vi "Demo Seq Tester.vi"() -> ()   [LabVIEW 2014]
uses:
  <vilib>/Utility/miscctls.llb/LVRowAndColumnTypeDef.ctl
  TypeDefs/STEP Display.ctl
  Mimico Display/TypeDefs/Mimic Data.ctl
  Mimico Display/TypeDefs/BG Image.ctl
  Mimico Display/TypeDefs/mObject.ctl
  SeqLoop/TypeDefs/Sequence.ctl
  SeqLoop/Classes/STEP/STEP.lvclass
  SeqLoop/TypeDefs/LogicParsedExpression.ctl
  SeqLoop/TypeDefs/HW InOut MAP.ctl
  SeqLoop/TypeDefs/Program.ctl
  APIs/Data Queue/Control Data Cluster.ctl
  SEQ Monitoring Global Variables.vi
  DO Monitoring Global Variables.vi
  APIs/Message Queue/Enqueue Message (Single).vi
  APIs/Message Queue/WINFAS 2 Message Queue.lvlib
  SeqLoop/SeqLoop.lvlib
  Mimico Display/Mimico Display.lvlib
  APIs/Data Queue/WINFAS 2 Data Queue.lvlib
panel:
  out "Current Prog Name":string caption="Info"
  out "Current Prog Info":string caption="Info"
  in  "MIMIC":bool
  in  "SEC":bool
  in  "HOME":bool
  in  "Tab Control":enum32{"HOME", "SEC", "MIMIC", "MESSAGE"}(tab)=enum."SEC"
  in  "New Cfg":bool
  in  "Open Cfg":bool
  in  "Save Cfg":bool
  in  "New Prog":bool
  in  "Delete Prog":bool
  in  "Config Prog":bool
  in  "I/O Config":bool
  in  "Editor de Programas":i32(listbox)=-1 caption="Secuencia"
  out "Current Sequence":string[][](table)
  in  "Angle":sgl(knob) scale=-720.0..720.0
  in  "Start Sec A-Z":bool
  in  "Start Sec Ciclo":bool
  in  "Tab Control HardW":enum32{"Hw 1", "Hw 2", "Hw 3", "Hw 4", "Hw 5"}(tab)
  in  "Conf In":T1
  in  "Conf In 2":T1
  in  "Conf In 3":T1
  in  "Conf In 4":T1
  in  "Conf In 5":T1
  in  "OutPuts":T2(tab)
  out "View Out":T3
  out "View Out 2":T3
  out "View Out 3":T3
  out "View Out 4":T3
  out "View Out 5":T3
  out "Error":bool
  out "Alarma":bool
  in  "Start Sec Special":bool
  out "Show Main Error&Alarm":string[][](table)
  out "Acept":bool
  out "Alarms Message":string
  out "Error Message":string
  out "Operator Message":string
  out "Mimic":picture
  out "MATH":string
  out "HWAsync 10":string
  out "HWAsync 9":string
  out "HWAsync 8":string
  out "HWAsync 7":string
  out "HWAsync 6":string
  out "HWAsync 5":string
  out "HWAsync 4":string
  out "HWAsync 3":string
  out "HWAsync 2":string
  out "HWAsync 1":string
  out "HWSync 5":string
  out "DO 5":bool[](array[boolean]) caption="DO-HWSync 5 -->"
  out "HWSync 4":string
  out "DO 4":bool[](array[boolean]) caption="DO-HWSync 4 -->"
  out "HWSync 3":string
  out "DO 3":bool[](array[boolean]) caption="DO-HWSync 3 -->"
  out "HWSync 2":string
  out "DO 2":bool[](array[boolean]) caption="DO-HWSync 2 -->"
  out "HWSync 1":string
  out "DO 1":bool[](array[boolean]) caption="DO-HWSync 1 -->"
  in  "MESSAGE":bool
  in  "error in (no error)":errorcluster
  in  "Tab Control 2":enum32{"HOME", "PIC", "TAB"}(tab)=enum."PIC"
  out "Mimic Small":picture
  out "Cond. Avan.":string[][](table)
  # "DEMO - Secuencial"
  # "Lista de Programas de Medición"
  # "Editor de Programas"
  # "Instrucciones: \n1)Utilice los botones de crear o borrar programa para agregar o borrar la referencia a la \"Lista de Programas de Medición\".\n2)Utilice la opción de configuración de programas para editar o configurar el programa previamente creado o cargado.\n3)Utilice la opción de configuración de I/O para configurar todas las entradas y salidas que se deseen usar."
  # "Configuración"
  # "Secuencia de Ciclo de Medición"
  # "Estado"
  # "Encoder"
  # "Mensaje de Operador:"
  # "Alarmas:"
  # "Dispositivos SINCRONOS"
  # "Módulo MATEMATICO"
  # "Dispositivos ASINCRONOS"
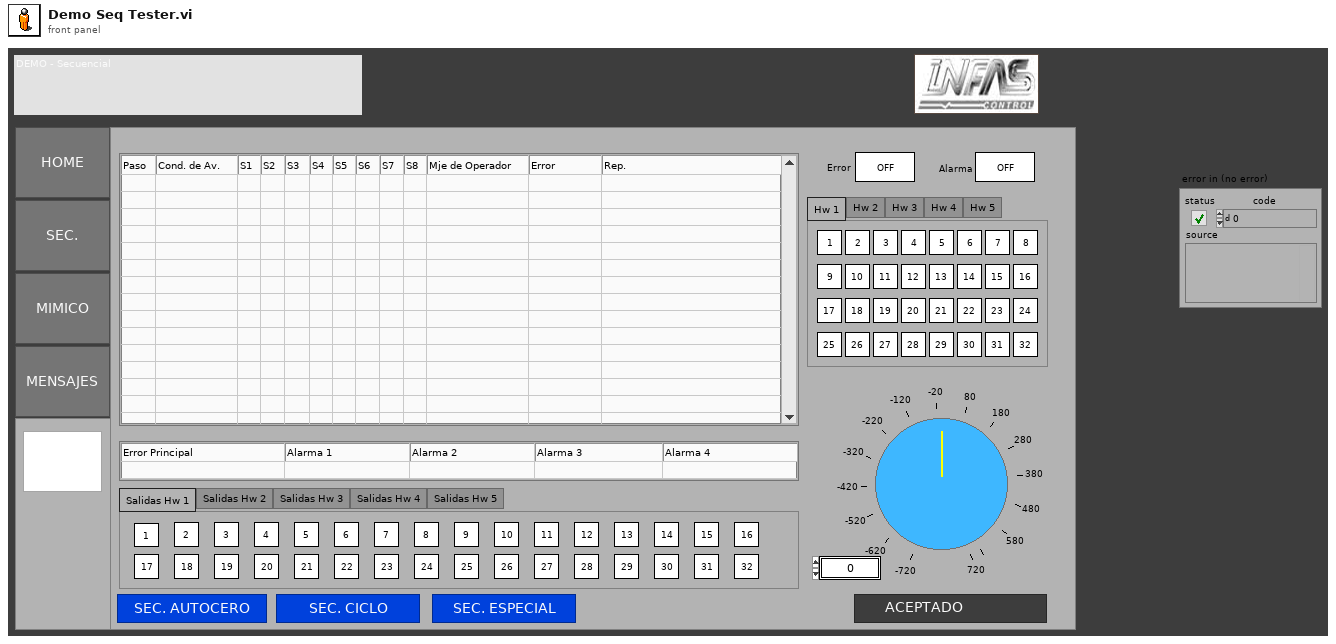
[diagram p1: front panel]
types:
  T1 = cluster{"Boolean 31":bool, "Boolean 2":bool, "Boolean 30":bool, "Boolean 29":bool, "Boolean 28":bool, "Boolean 27":bool, "Boolean 13":bool, "Boolean 14":bool, "Boolean 26":bool, "Boolean 25":bool, "Boolean 24":bool, "Boolean 23":bool, "Boolean 32":bool, "Boolean 1":bool, "Boolean 3":bool, "Boolean 4":bool, "Boolean 5":bool, "Boolean 6":bool, "Boolean 7":bool, "Boolean 8":bool, "Boolean 9":bool, "Boolean 10":bool, "Boolean 11":bool, "Boolean 12":bool, "Boolean 20":bool, "Boolean 18":bool, "Boolean 19":bool, "Boolean 17":bool, "Boolean 16":bool, "Boolean 15":bool, "Boolean 22":bool, "Boolean 21":bool}
  T2 = enum32{"Salidas Hw 1", "Salidas Hw 2", "Salidas Hw 3", "Salidas Hw 4", "Salidas Hw 5"}
  T3 = cluster{"Boolean 36":bool, "Boolean 3":bool, "Boolean 35":bool, "Boolean 34":bool, "Boolean 33":bool, "Boolean 32":bool, "Boolean 16":bool, "Boolean 17":bool, "Boolean 26":bool, "Boolean 25":bool, "Boolean 24":bool, "Boolean 23":bool, "Boolean 37":bool, "Boolean 1":bool, "Boolean 15":bool, "Boolean 4":bool, "Boolean 5":bool, "Boolean 6":bool, "Boolean 7":bool, "Boolean 8":bool, "Boolean 9":bool, "Boolean 10":bool, "Boolean 11":bool, "Boolean 12":bool, "Boolean 38":bool, "Boolean 21":bool, "Boolean 22":bool, "Boolean 20":bool, "Boolean 19":bool, "Boolean 18":bool, "Boolean 40":bool, "Boolean 39":bool}
  T4 = typedef "SeqLoop.lvlib/Sequence.ctl" = cluster{"STEPs":refnum<class "STEP.lvclass">[], "Main Error&Alarm":cluster{"Main Error":T5, "Main Alarm 1":T5, "Main Alarm 2":T5, "Main Alarm 3":T5, "Main Alarm 4":T5}, "STEP Type":refnum<class "STEP.lvclass">}
  T5 = typedef "SeqLoop.lvlib/LogicParsedExpression.ctl" = cluster{"RPN ":string[], "Variables":string[], "Ctes":string[], "Formula":string, "Message":string}
  T6 = cluster{"HWS1":string, "HWS2":string, "HWS3":string, "HWS4":string, "HWS5":string, "MATH":string}
  T7 = enum8{"Enabled", "Disabled", "Disabled and Grayed Out"}
  T8 = typedef "STEP Display.ctl" = cluster{"Mimic Data":T9, "Operator Mssg":string, "Error":cluster{"true?":bool, "Message":string}, "Alarm 1":cluster{"true?":bool, "Message":string}, "Alarm 2":cluster{"true?":bool, "Message":string}, "Alarm 3":cluster{"true?":bool, "Message":string}, "Alarm 4":cluster{"true?":bool, "Message":string}}
  T9 = typedef "SeqLoop.lvlib/Mimico Display.lvlib/Mimic Data.ctl" = cluster{"BG Image":T10, "Mimic mObjects":T11[]}
  T10 = typedef "SeqLoop.lvlib/Mimico Display.lvlib/BG Image.ctl" = cluster{"Path":path, "point":cluster{"x":i16, "y":i16}}
  T11 = typedef "SeqLoop.lvlib/Mimico Display.lvlib/mObject.ctl" = cluster{"point":cluster{"x":i16, "y":i16}, "Precision (Digits)":i32, "Visible?":bool, "Ref":string, "Comment":string}
  T12 = cluster{"File Direction":path, "Progs Data":variant}
  T13 = typedef "LVRowAndColumnTypeDef.ctl" = cluster{"Row":i32, "Column":i32}
  T14 = typedef "WINFAS 2 Data Queue.lvlib/All Data Queues Cluster.ctl" = cluster{"Queues":cluster{"ACQ HWSync1":refnum<queue>, "ACQ HWSync2":refnum<queue>, "ACQ HWSync3":refnum<queue>, "ACQ HWSync4":refnum<queue>, "ACQ HWSync5":refnum<queue>}, "Notifiers":cluster{"Control":cluster{"CTRL HWSync1":refnum<notifier>, "CTRL HWSync2":refnum<notifier>, "CTRL HWSync3":refnum<notifier>, "CTRL HWSync4":refnum<notifier>, "CTRL HWSync5":refnum<notifier>}, "Acquisition":cluster{"ACQ HWSync1":refnum<notifier>, "ACQ HWSync2":refnum<notifier>, "ACQ HWSync3":refnum<notifier>, "ACQ HWSync4":refnum<notifier>, "ACQ HWSync5":refnum<notifier>}, "Async":cluster{"ACQ HWAsync1":refnum<notifier>, "ACQ HWAsync2":refnum<notifier>, "ACQ HWAsync3":refnum<notifier>, "ACQ HWAsync4":refnum<notifier>, "ACQ HWAsync5":refnum<notifier>, "ACQ HWAsync6":refnum<notifier>, "ACQ HWAsync7":refnum<notifier>, "ACQ HWAsync8":refnum<notifier>, "ACQ HWAsync9":refnum<notifier>, "ACQ HWAsync10":refnum<notifier>}}}
  T15 = typedef "WINFAS 2 Message Queue.lvlib/All Message Queues.ctl" = cluster{"CORE":refnum<queue>, "Event UI":refnum<queue>, "Display UI":refnum<queue>, "MATH":refnum<queue>, "SEQ":refnum<queue>, "DB":refnum<queue>, "ERR":refnum<queue>, "HAL":refnum<queue>, "HWSync1":refnum<queue>, "HWSync2":refnum<queue>, "HWSync3":refnum<queue>, "HWSync4":refnum<queue>, "HWSync5":refnum<queue>, "HWAsync1":refnum<queue>, "HWAsync2":refnum<queue>, "HWAsync3":refnum<queue>, "HWAsync4":refnum<queue>, "HWAsync5":refnum<queue>, "HWAsync6":refnum<queue>, "HWAsync7":refnum<queue>, "HWAsync8":refnum<queue>, "HWAsync9":refnum<queue>, "HWAsync10":refnum<queue>}
  T16 = cluster{"CTRL HWSync1":refnum<notifier>, "CTRL HWSync2":refnum<notifier>, "CTRL HWSync3":refnum<notifier>, "CTRL HWSync4":refnum<notifier>, "CTRL HWSync5":refnum<notifier>}
  T17 = cluster{"File Direction":path, "Progs Data":variant}[]
  T18 = enum16{"open", "replace", "create", "open or create", "replace or create", "replace or create with confirmation"}
  T19 = typedef "SeqLoop.lvlib/HW InOut MAP.ctl" = cluster{"Inputs":cluster{"Entrada":i32, "Descripción":string, "Habilitada?":bool}[][], "Outputs":cluster{"Salida":i32, "Descripción":string, "Habilitada?":bool, "Formula":string, "Tipo de Salida":string}[][]}
  T20 = typedef "SeqLoop.lvlib/Program.ctl" = cluster{"Prog. Data":cluster{"Tipo de Programa":string, "Operación":i32, "Pieza":i32, "Descripción":string, "Nombre Programa":string, "Autor":string, "Cód. Prog.":i32, "Diseño":string, "Total Meds.:":i32, "Total Meds. Aux.:":i32}, "All Sequences":cluster{"Measurement":T4, "AutoZero":T4, "Special":T4}}
  T21 = cluster{cluster{"File Direction":path, "Progs Data":variant}[]}
  T22 = cluster{"Progs":cluster{"File Direction":path, "Progs Data":variant}, "Program Type":string}
  T23 = typedef "WINFAS 2 Data Queue.lvlib/Control Data Cluster.ctl" = cluster{"Encoder":sgl, "DI":bool[], "DO":bool[]}
  T24 = cluster{"format string":string, "Measurement Index":i32[]}
  T25 = cluster{"MAX(T) or MIN (F)?":bool, "Mastering TDX Index":i32[]}
  T26 = cluster{"Main Error":T5, "Main Alarm 1":T5, "Main Alarm 2":T5, "Main Alarm 3":T5, "Main Alarm 4":T5}
  T27 = enum32{"invalid app kind", "Development System", "Run Time System", "Student Edition", "Embedded LabVIEW", "Evaluation", "Custom"}
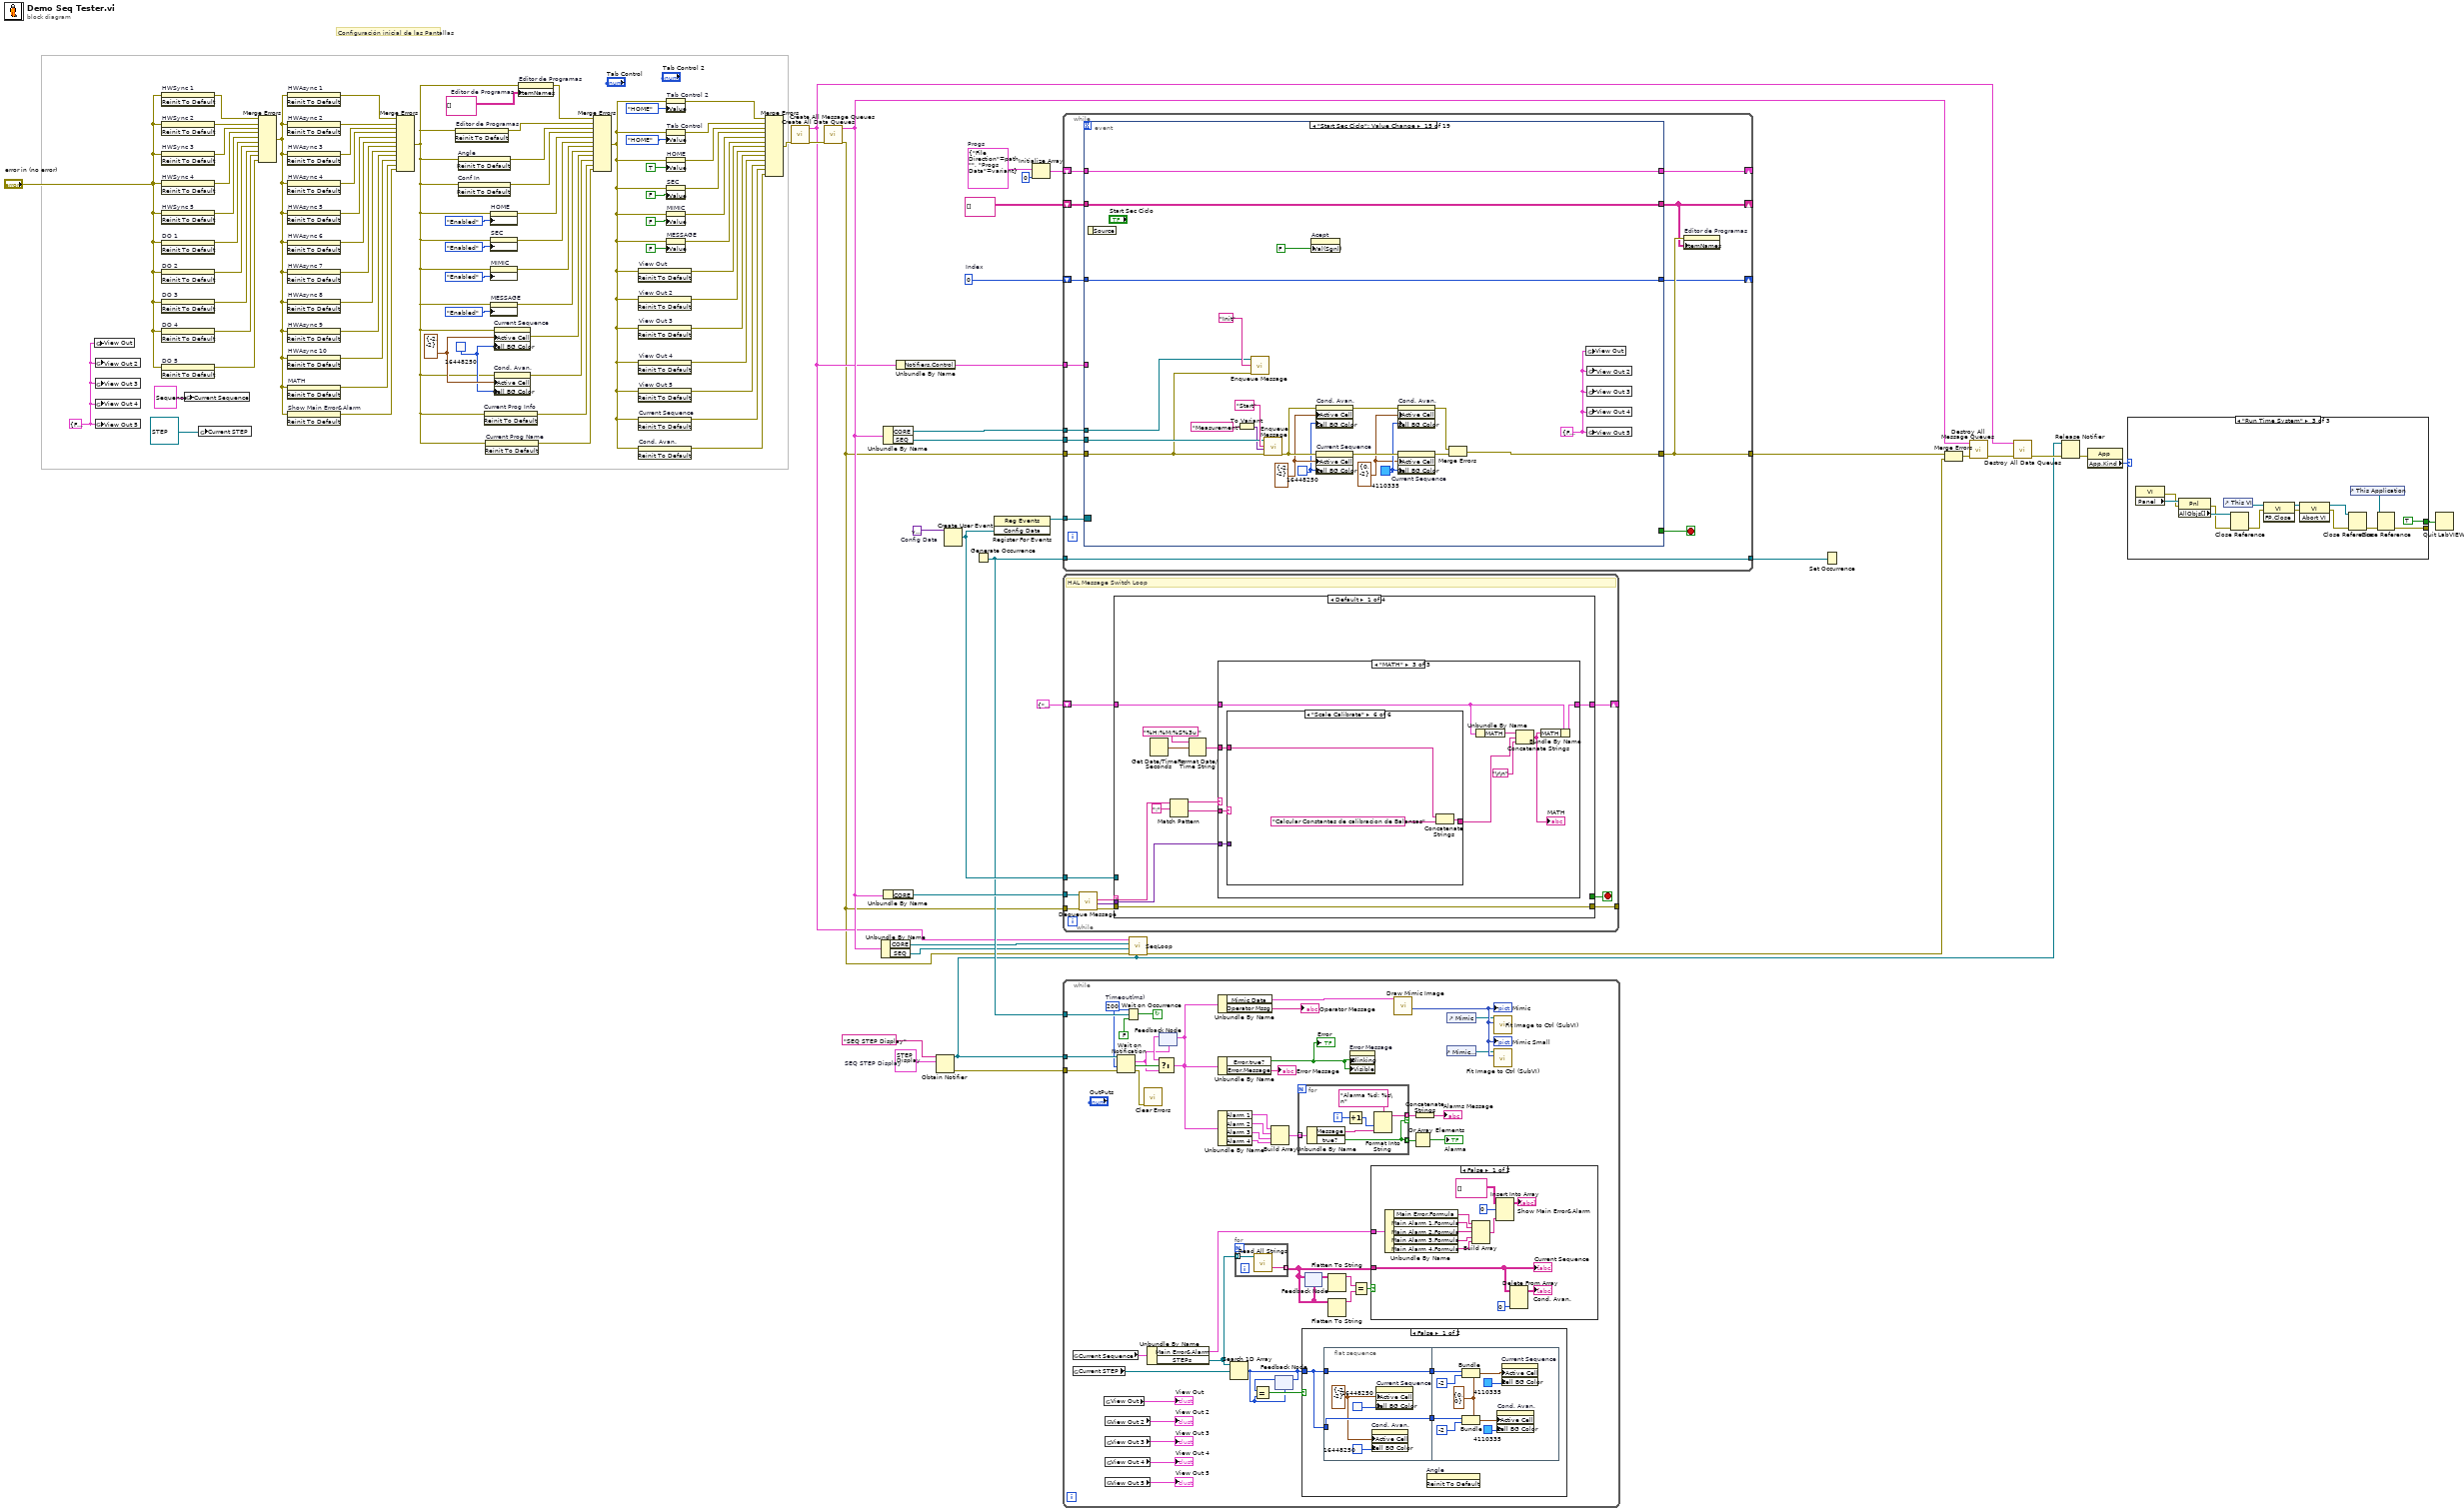
[diagram p0: block diagram]
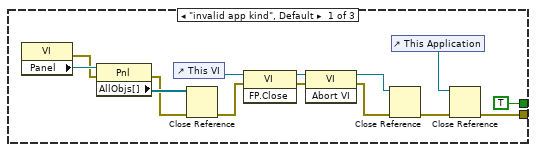
[diagram p4: hidden frame]
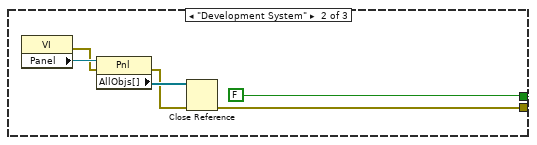
[diagram p5: hidden frame]
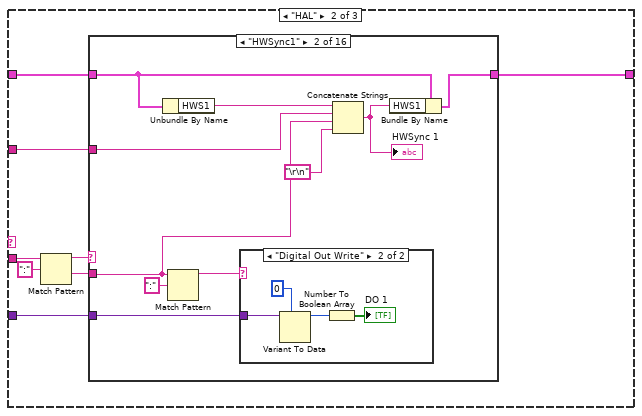
[diagram p7: hidden frame]
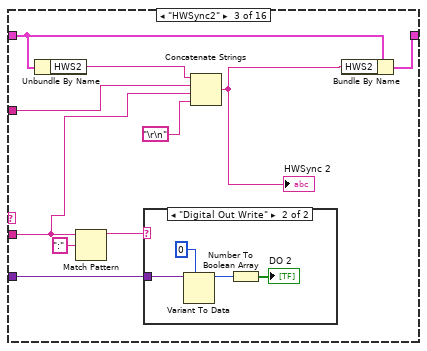
[diagram p10: hidden frame]
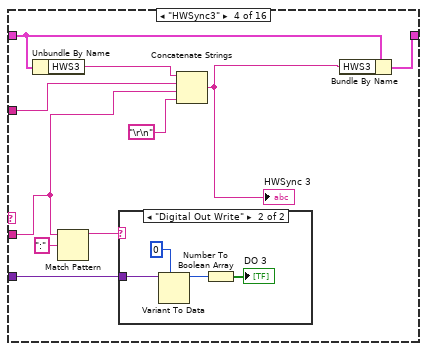
[diagram p12: hidden frame]
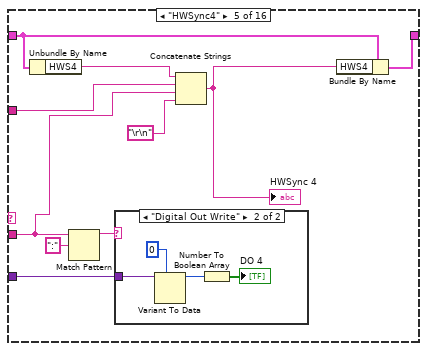
[diagram p14: hidden frame]
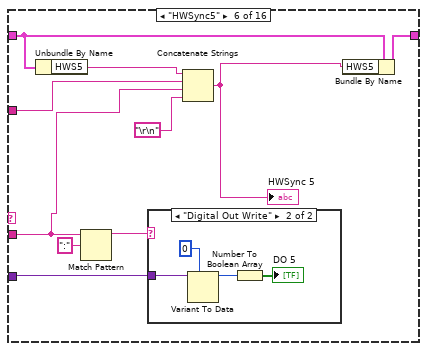
[diagram p16: hidden frame]
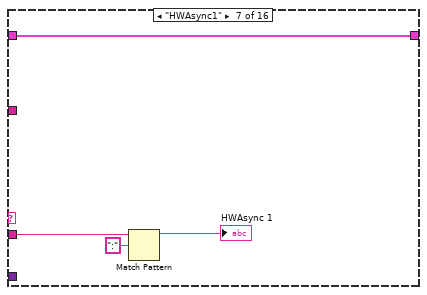
[diagram p18: hidden frame]
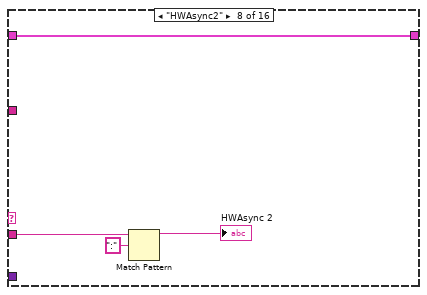
[diagram p19: hidden frame]
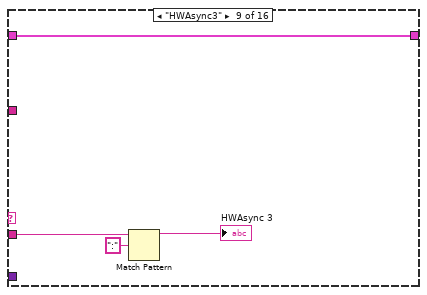
[diagram p20: hidden frame]
diagram:
  w1 = T3 {"Boolean 36"=FALSE, "Boolean 3"=FALSE, "Boolean 35"=FALSE, "Boolean 34"=FALSE, "Boolean 33"=FALSE, "Boolean 32"=FALSE, "Boolean 16"=FALSE, "Boolean 17"=FALSE, "Boolean 26"=FALSE, "Boolean 25"=FALSE, "Boolean 24"=FALSE, "Boolean 23"=FALSE, "Boolean 37"=FALSE, "Boolean 1"=FALSE, "Boolean 15"=FALSE, "Boolean 4"=FALSE, "Boolean 5"=FALSE, "Boolean 6"=FALSE, "Boolean 7"=FALSE, "Boolean 8"=FALSE, "Boolean 9"=FALSE, "Boolean 10"=FALSE, "Boolean 11"=FALSE, "Boolean 12"=FALSE, "Boolean 38"=FALSE, "Boolean 21"=FALSE, "Boolean 22"=FALSE, "Boolean 20"=FALSE, "Boolean 19"=FALSE, "Boolean 18"=FALSE, "Boolean 40"=FALSE, "Boolean 39"=FALSE} ("View Out")
  w52 = T8 {"Mimic Data"={"BG Image"={"Path"=path "", "point"={"x"=0, "y"=0}}, "Mimic mObjects"=[]}, "Operator Mssg"="", "Error"={"true?"=FALSE, "Message"=""}, "Alarm 1"={"true?"=FALSE, "Message"=""}, "Alarm 2"={"true?"=FALSE, "Message"=""}, "Alarm 3"={"true?"=FALSE, "Message"=""}, "Alarm 4"={"true?"=FALSE, "Message"=""}}  # SEQ STEP Display
  w70 = T12 {"File Direction"=path "", "Progs Data"=variant}  # Progs
  w44 = T13 {"Row"=-2, "Column"=-2} ("Active Cell:Active Cell")
  w43 = u32 16448250
  w73 = string[][] []  # Editor de Programas
  w87 = 0  # Index
  w96 = variant  # Config Data
  # "Configuración inicial de las Pantallas"
  n1 = global write "DO Monitoring Global Variables.vi" "View Out"(w1) -> ()
  n2 = global write "DO Monitoring Global Variables.vi" "View Out 2"(w1) -> ()
  n3 = global write "DO Monitoring Global Variables.vi" "View Out 3"(w1) -> ()
  n4 = global write "DO Monitoring Global Variables.vi" "View Out 4"(w1) -> ()
  n5 = global write "DO Monitoring Global Variables.vi" "View Out 5"(w1) -> ()
  n6 = invoke on="HWSync 1" class="Str" method="Reinit To Default"(error in="error in (no error)") -> (error out=w22:errorcluster)  [unwired: 2 in, 2 out]
  n7 = invoke on="HWSync 2" class="Str" method="Reinit To Default"(error in="error in (no error)") -> (error out=w21:errorcluster)  [unwired: 2 in, 2 out]
  n8 = invoke on="HWSync 3" class="Str" method="Reinit To Default"(error in="error in (no error)") -> (error out=w20:errorcluster)  [unwired: 2 in, 2 out]
  n9 = invoke on="HWSync 4" class="Str" method="Reinit To Default"(error in="error in (no error)") -> (error out=w19:errorcluster)  [unwired: 2 in, 2 out]
  n10 = invoke on="HWSync 5" class="Str" method="Reinit To Default"(error in="error in (no error)") -> (error out=w18:errorcluster)  [unwired: 2 in, 2 out]
  n11 = invoke on="DO 1" class="Arr (strict)" method="Reinit To Default"(error in="error in (no error)") -> (error out=w17:errorcluster)  [unwired: 2 in, 2 out]
  n12 = invoke on="DO 2" class="Arr (strict)" method="Reinit To Default"(error in="error in (no error)") -> (error out=w16:errorcluster)  [unwired: 2 in, 2 out]
  n13 = invoke on="DO 3" class="Arr (strict)" method="Reinit To Default"(error in="error in (no error)") -> (error out=w15:errorcluster)  [unwired: 2 in, 2 out]
  n14 = invoke on="DO 4" class="Arr (strict)" method="Reinit To Default"(error in="error in (no error)") -> (error out=w14:errorcluster)  [unwired: 2 in, 2 out]
  n15 = invoke on="DO 5" class="Arr (strict)" method="Reinit To Default"(error in="error in (no error)") -> (error out=w13:errorcluster)  [unwired: 2 in, 2 out]
  n16 = global write "SEQ Monitoring Global Variables.vi" "Current Sequence"(T4 {"STEPs"=[], "Main Error&Alarm"={"Main Error"={"RPN "=[], "Variables"=[], "Ctes"=[], "Formula"="", "Message"=""}, "Main Alarm 1"={"RPN "=[], "Variables"=[], "Ctes"=[], "Formula"="", "Message"=""}, "Main Alarm 2"={"RPN "=[], "Variables"=[], "Ctes"=[], "Formula"="", "Message"=""}, "Main Alarm 3"={"RPN "=[], "Variables"=[], "Ctes"=[], "Formula"="", "Message"=""}, "Main Alarm 4"={"RPN "=[], "Variables"=[], "Ctes"=[], "Formula"="", "Message"=""}}, "STEP Type"=refnum} ("Current Sequence")) -> ()
  n17 = global write "SEQ Monitoring Global Variables.vi" "Current STEP"(refnum<class "STEP.lvclass"> refnum ("Current STEP")) -> ()
  n18 = Merge Errors(w22, w21, w20, w19, w18, w17, w16, w15, w14, w13) -> (w3:errorcluster)
  n19 = invoke on="HWAsync 1" class="Str" method="Reinit To Default"(error in=w3) -> (error out=w33:errorcluster)  [unwired: 2 in, 2 out]
  n20 = invoke on="HWAsync 2" class="Str" method="Reinit To Default"(error in=w3) -> (error out=w32:errorcluster)  [unwired: 2 in, 2 out]
  n21 = invoke on="HWAsync 3" class="Str" method="Reinit To Default"(error in=w3) -> (error out=w31:errorcluster)  [unwired: 2 in, 2 out]
  n22 = invoke on="HWAsync 4" class="Str" method="Reinit To Default"(error in=w3) -> (error out=w30:errorcluster)  [unwired: 2 in, 2 out]
  n23 = invoke on="HWAsync 5" class="Str" method="Reinit To Default"(error in=w3) -> (error out=w29:errorcluster)  [unwired: 2 in, 2 out]
  n24 = invoke on="HWAsync 6" class="Str" method="Reinit To Default"(error in=w3) -> (error out=w28:errorcluster)  [unwired: 2 in, 2 out]
  n25 = invoke on="HWAsync 7" class="Str" method="Reinit To Default"(error in=w3) -> (error out=w27:errorcluster)  [unwired: 2 in, 2 out]
  n26 = invoke on="HWAsync 8" class="Str" method="Reinit To Default"(error in=w3) -> (error out=w26:errorcluster)  [unwired: 2 in, 2 out]
  n27 = invoke on="HWAsync 9" class="Str" method="Reinit To Default"(error in=w3) -> (error out=w25:errorcluster)  [unwired: 2 in, 2 out]
  n28 = invoke on="HWAsync 10" class="Str" method="Reinit To Default"(error in=w3) -> (error out=w24:errorcluster)  [unwired: 2 in, 2 out]
  n29 = invoke on="MATH" class="Str" method="Reinit To Default"(error in=w3) -> (error out=w23:errorcluster)  [unwired: 2 in, 2 out]
  n30 = invoke on="Show Main Error&Alarm" class="Tbl (strict)" method="Reinit To Default"(error in=w3) -> (error out=w4:errorcluster)  [unwired: 2 in, 2 out]
  n31 = Merge Errors(w33, w32, w31, w30, w29, w28, w27, w26, w25, w24, w23, w4) -> (w11:errorcluster)
  n32 = invoke on="Editor de Programas" class="MCListbox (strict)" method="Reinit To Default"(error in=w11) -> (error out=w54:errorcluster)  [unwired: 2 in, 2 out]
  n33 = invoke on="Angle" class="Knob (strict)" method="Reinit To Default"(error in=w11) -> (error out=w99:errorcluster)  [unwired: 2 in, 2 out]
  n34 = invoke on="Conf In" class="Clust (strict)" method="Reinit To Default"(error in=w11) -> (error out=w100:errorcluster)  [unwired: 2 in, 2 out]
  n35 = invoke on="Current Prog Info" class="Str" method="Reinit To Default"(error in=w11) -> (error out=w39:errorcluster)  [unwired: 2 in, 2 out]
  n36 = invoke on="Current Prog Name" class="Str" method="Reinit To Default"(error in=w11) -> (error out=w10:errorcluster)  [unwired: 2 in, 2 out]
  n37 = property on="HOME" class="Bool (strict)"(error in=w11, "DisabledEnum"=T7."Enabled" ("Disabled")) -> (error out=w77:errorcluster)  [unwired: 1 in, 1 out]
  n38 = property on="SEC" class="Bool (strict)"(error in=w11, "DisabledEnum"=T7."Enabled" ("Disabled")) -> (error out=w68:errorcluster)  [unwired: 1 in, 1 out]
  n39 = property on="MIMIC" class="Bool (strict)"(error in=w11, "DisabledEnum"=T7."Enabled" ("Disabled")) -> (error out=w67:errorcluster)  [unwired: 1 in, 1 out]
  n40 = property on="MESSAGE" class="Bool (strict)"(error in=w11, "DisabledEnum"=T7."Enabled" ("Disabled")) -> (error out=w45:errorcluster)  [unwired: 1 in, 1 out]
  n41 = property on="Current Sequence" class="Tbl (strict)"(error in=w11, "Active Cell"=w44, "Cell BG Color"=w43) -> (error out=w46:errorcluster)  [unwired: 1 in, 1 out]
  n42 = property on="Cond. Avan." class="Tbl (strict)"(error in=w11, "Active Cell"=w44, "Cell BG Color"=w43) -> (error out=w42:errorcluster)  [unwired: 1 in, 1 out]
  n43 = property on="Editor de Programas" class="MCListbox (strict)"(error in=w11, "ItemNames"=w73) -> (error out=w53:errorcluster)  [unwired: 1 in, 1 out]
  n44 = Merge Errors(w53, w54, w99, w100, w77, w68, w67, w45, w46, w42, w39, w10) -> (w9:errorcluster)
  n45 = invoke on="View Out" class="Clust (strict)" method="Reinit To Default"(error in=w9) -> (error out=w38:errorcluster)  [unwired: 2 in, 2 out]
  n46 = invoke on="View Out 2" class="Clust (strict)" method="Reinit To Default"(error in=w9) -> (error out=w37:errorcluster)  [unwired: 2 in, 2 out]
  n47 = invoke on="View Out 3" class="Clust (strict)" method="Reinit To Default"(error in=w9) -> (error out=w36:errorcluster)  [unwired: 2 in, 2 out]
  n48 = invoke on="View Out 4" class="Clust (strict)" method="Reinit To Default"(error in=w9) -> (error out=w35:errorcluster)  [unwired: 2 in, 2 out]
  n49 = invoke on="View Out 5" class="Clust (strict)" method="Reinit To Default"(error in=w9) -> (error out=w34:errorcluster)  [unwired: 2 in, 2 out]
  n50 = invoke on="Current Sequence" class="Tbl (strict)" method="Reinit To Default"(error in=w9) -> (error out=w8:errorcluster)  [unwired: 2 in, 2 out]
  n51 = invoke on="Cond. Avan." class="Tbl (strict)" method="Reinit To Default"(error in=w9) -> (error out=w7:errorcluster)  [unwired: 2 in, 2 out]
  n52 = property on="Tab Control 2" class="TabCtl (strict)"(error in=w9, "Value"=enum32{"HOME", "PIC", "TAB"}."HOME" ("Tab Control 2")) -> (error out=w41:errorcluster)  [unwired: 1 in, 1 out]
  n53 = property on="Tab Control" class="TabCtl (strict)"(error in=w9, "Value"=enum32{"HOME", "SEC", "MIMIC", "MESSAGE"}."HOME" ("Tab Control")) -> (error out=w76:errorcluster)  [unwired: 1 in, 1 out]
  n54 = property on="HOME" class="Bool (strict)"(error in=w9, "Value"=TRUE ("HOME")) -> (error out=w75:errorcluster)  [unwired: 1 in, 1 out]
  n55 = property on="SEC" class="Bool (strict)"(error in=w9, "Value"=FALSE ("CICLO")) -> (error out=w74:errorcluster)  [unwired: 1 in, 1 out]
  n56 = property on="MIMIC" class="Bool (strict)"(error in=w9, "Value"=FALSE ("CONFIG.")) -> (error out=w66:errorcluster)  [unwired: 1 in, 1 out]
  n57 = property on="MESSAGE" class="Bool (strict)"(error in=w9, "Value"=FALSE ("CONFIG.")) -> (error out=w49:errorcluster)  [unwired: 1 in, 1 out]
  n58 = Merge Errors(w41, w76, w75, w74, w66, w49, w38, w37, w36, w35, w34, w8, w7) -> (w65:errorcluster)
  n59 = call "Create All Data Queues.vi"("Error In"=w65) -> ("Error Out"=w64:errorcluster, "WINFAS 2 Data Queue.lvlib:All Data Queues Cluster"=w57:T14)  [unwired: 9 in]
  n60 = call "Create All Message Queues.vi"("error in (no error)"=w64) -> ("error out"=w56:errorcluster, "Message Queues Out"=w61:T15)  [unwired: 9 in]
  n61 = Unbundle By Name(w61) -> ("CORE"=w59:refnum<queue>, "SEQ"=w58:refnum<queue>)
  n62 = Unbundle By Name(w61) -> ("CORE"=w92:refnum<queue>, "SEQ"=w93:refnum<queue>)
  n63 = Unbundle By Name(w61) -> ("CORE"=w97:refnum<queue>)
  n64 = Unbundle By Name(w57) -> ("Notifiers.Control"=w60:T16)
  n65 = Obtain Notifier(name (unnamed)="SEQ STEP Display", notification data type=w52) -> (notifier out=w51:refnum<notifier>, error out=w83:errorcluster)  [unwired: 2 in, 1 out]
  n66 = Create User Event(user event datatype=w96) -> (user event=w94:refnum<user-event>)  [unwired: 1 in, 1 out]
  n67 = Generate Occurrence() -> (w81:refnum<k4>)
  n68 = register-events(w94) -> (reference out=w95:refnum<event-registration>)  [unwired: 2 in, 1 out]
  n69 = Initialize Array(w70, 0 ("dimension size")) -> (w71:T17)
  n70 = while {
    tunnel: w56 -> [w115]
    tunnel: [w109] -> w101
    tunnel: w95 -> [w113]
    tunnel: w93 -> [w112]
    tunnel: w92 -> [w111]
    shift-right: [w108] -> _
    shift-left: w87 -> [w110]
    tunnel: w81 -> [w107]
    tunnel: [w107] -> w82
    shift-right: [w105] -> _
    shift-left: w71 -> [w106]
    shift-right: [w103] -> _
    shift-left: string[][] [] -> [w104]
    tunnel: w60 -> [w102]
    stop <- w114 stop-if-true
    n71 = event shown="[14] \"Start Sec Ciclo\": Value Change" {
      selector: w113 -> [_ _ _ _ _ _ _ _ _ _ _ _ _ _ _ _ _ _ _]
      dyn-events: _ -> [_ _ _ _ _ _ _ _ _ _ _ _ _ _ _ _ _ _ _]
      timeout: _ -> [_ _ _ _ _ _ _ _ _ _ _ _ _ _ _ _ _ _ _]
      tunnel: w115 -> [w132 w146 w168 w207 w256 w286 w311 w334 w362 w387 w409 w424 w430 w457 w479 w501 w522 w563 w591]
      tunnel: [w137 w142 w184 w205 w255 w306 w327 w359 w381 w394 w407 w425 w447 w455 w477 w499 w520 w557 w589] -> w109
      tunnel: [_ _ _ _ _ _ _ _ _ _ _ _ _ _ _ _ _ _ TRUE ("Discard?")] -> w114
      tunnel: w112 -> [w139 _ w169 w208 _ w284 _ _ _ _ w410 w423 _ w474 w495 w517 _ _ w587]
      tunnel: w111 -> [_ _ _ _ _ _ _ _ _ _ _ _ _ w456 w478 w500 _ _ w588]
      tunnel: ["Editor de Programas" w149 w172 w218 _ w290 w323 w338 w379 _ w412 w420 w442 w472 w494 w516 w519 w581 w586] -> w108
      tunnel: w110 -> [_ w151 w175 w218 _ w278 w323 w338 w379 _ w412 w420 w442 w472 w494 w516 w519 w581 w586]
      tunnel: w106 -> [w141 w145 w177 w209 w258 w279 w322 w352 w375 w406 w411 w422 w449 w471 w493 w515 w525 w583 w585]
      tunnel: [w141 w144 w176 w206 w258 w291 w322 w352 w375 w406 w411 w422 w448 w471 w493 w515 w525 w583 w585] -> w105
      tunnel: w104 -> [w116 w148 w174 w203 w257 w307 w321 w339 w371 w405 w416 w421 w445 w470 w492 w514 w524 w582 w584]
      tunnel: [w116 w147 w173 w204 w257 w308 w321 w339 w371 w405 w416 w421 w444 w470 w492 w514 w524 w582 w584] -> w103
      tunnel: w102 -> [_ _ _ _ _ _ _ _ _ _ _ _ _ _ _ _ _ w556 _]
      event "Editor de Programas": Value Change {
        w131 = T13 {"Row"=-2, "Column"=-2} ("Active Cell:Active Cell")
        w130 = u32 16448250
        n72 = event-data() -> ()  [unwired: 1 in, 1 out]
        n73 = property on="Current Sequence" class="Tbl (strict)"(error in=w132, "Active Cell"=w131, "Cell BG Color"=w130) -> (error out=w128:errorcluster)  [unwired: 1 in, 1 out]
        n74 = property on="Cond. Avan." class="Tbl (strict)"(error in=w132, "Active Cell"=w131, "Cell BG Color"=w130) -> (error out=w129:errorcluster)  [unwired: 1 in, 1 out]
        n75 = Index Array(array=w116, index (row) #1="Editor de Programas", index (col) #1=1 ("disabled index (col)"), index (row) #2="Editor de Programas", index (col) #2=0 ("disabled index (col)"), index (row) #3="Editor de Programas", index (col) #3=2 ("index (row)"), index (row) #4="Editor de Programas", index (col) #4=6 ("index (col)")) -> (element #1=w119:string, element #2=w126:string, element #3=w125:string, element #4=w124:string)
        n76 = Merge Errors(w128, w129) -> (w127:errorcluster)
        n77 = Index Array(array=w141, index="Editor de Programas") -> (element=w138:T12)
        n78 = Unbundle By Name(w138) -> ("Progs Data"=w133:variant)
        n79 = Concatenate Strings("Nombre Programa: ", w119) -> (→"Current Prog Name":string)
        n80 = call-poly "Enqueue Message.vi"("error in (no error)"=w127, "Message Data"=w133, "Message"="Config:Set" ("Cmd String"), "Message Queue"=w139) -> ("error out"=w137:errorcluster)  [unwired: 6 in, 1 out]
        n81 = Format Into String(format string="COD. Prog. : %s - Descripción: %s - Tipo de Prog.: %s", w126, w125, w124) -> (resulting string=→"Current Prog Info":string)  [unwired: 2 in, 1 out]
      }
      event "Delete Prog": Value Change {
        n82 = event-data() -> ()  [unwired: 1 in, 1 out]
        n83 = Increment(x=w151) -> (x+1=w152:i32)
        n84 = Number To Decimal String(number=w152) -> (decimal integer string=w154:string)  [unwired: 1 in]
        n85 = Concatenate Strings("Desea Borrar el elemento: " ("message"), w154) -> (w153:string)
        n86 = Two Button Dialog(message=w153) -> (T button?=w150:bool)  [unwired: 2 in]
        n87 = case shown="True" w150 {
          tunnel: [w159 w165] -> w147
          tunnel: w148 -> [w159 w164]
          tunnel: w151 -> [w158 w160]
          tunnel: w146 -> [w157 w163]
          tunnel: [w157 w163] -> w143
          tunnel: [w158 w160] -> w149
          tunnel: w145 -> [w156 w162]
          tunnel: [w156 w161] -> w144
          frame False {
          }
          frame True {
            n88 = Delete From Array(array=w162, index=w160) -> (array with subset deleted=w161:T17)  [unwired: 1 in, 1 out]
            n89 = Delete From Array(array=w164, index (row)=w160) -> (array with subset deleted=w165:string[][])  [unwired: 2 in, 1 out]
          }
        }
        n90 = invoke on="Current Prog Info" class="Str" method="Reinit To Default"(error in=w143) -> (error out=w142:errorcluster)  [unwired: 2 in, 2 out]
      }
      event "New Cfg": Value Change {
        w171 = T12 {"File Direction"=path "", "Progs Data"=variant}  # Progs
        n91 = event-data() -> ()  [unwired: 1 in, 1 out]
        n92 = Initialize Array(w171, 15 ("dimension size")) -> (w180:T17)
        n93 = Flatten To String(anything=w180) -> (data string=w182:string)  [unwired: 3 in, 2 out]
        n94 = Flatten To String(anything=w177) -> (data string=w181:string)  [unwired: 3 in, 2 out]
        n95 = Not Equal?(x=w181, y=w182) -> (x != y?=w183:bool)
        n96 = case "Algún Prog cargado?" shown="True" w183 {
          tunnel: [TRUE ("T button?") w189] -> w178
          frame False {
          }
          frame True {
            n97 = Two Button Dialog(message="Desea crear una nueva lista de Programas?\n(Se descargarán todos los Programas cargados)") -> (T button?=w189:bool)  [unwired: 2 in]
          }
        }
        n98 = case shown="True" w178 {
          tunnel: [w193 w201] -> w176
          tunnel: w177 -> [w193 _]
          tunnel: w175 -> [w191 _]
          tunnel: w174 -> [w192 _]
          tunnel: [w192 string[][] []] -> w173
          tunnel: [w191 0 ("Index")] -> w172
          tunnel: w169 -> [_ w196]
          tunnel: w168 -> [w190 w195]
          tunnel: [w190 w194] -> w166
          frame False {
          }
          frame True {
            w198 = T12 {"File Direction"=path "", "Progs Data"=variant}  # Progs
            n99 = call-poly "Enqueue Message.vi"("error in (no error)"=w195, "Message"="INIT" ("Cmd String"), "Message Queue"=w196) -> ("error out"=w194:errorcluster)  [unwired: 7 in, 1 out]
            n100 = Initialize Array(w198, 0 ("dimension size")) -> (w201:T17)
          }
        }
        n101 = invoke on="Angle" class="Knob (strict)" method="Reinit To Default"(error in=w166) -> (error out=w185:errorcluster)  [unwired: 2 in, 2 out]
        n102 = invoke on="Conf In" class="Clust (strict)" method="Reinit To Default"(error in=w166) -> (error out=w186:errorcluster)  [unwired: 2 in, 2 out]
        n103 = invoke on="Current Sequence" class="Tbl (strict)" method="Reinit To Default"(error in=w166) -> (error out=w170:errorcluster)  [unwired: 2 in, 2 out]
        n104 = invoke on="Cond. Avan." class="Tbl (strict)" method="Reinit To Default"(error in=w166) -> (error out=w167:errorcluster)  [unwired: 2 in, 2 out]
        n105 = Merge Errors(w185, w186, w170, w167) -> (w184:errorcluster)
      }
      event "Open Cfg": Value Change {
        n106 = event-data() -> ()  [unwired: 1 in, 1 out]
        n107 = call <vilib>:"Application Directory.vi"() -> ("Application Directory"=w214:path)
        n108 = Build Path(base path=w214, name or relative path="Configuraciones") -> (appended path=w215:path)
        n109 = call "File Dialog"("start path"=w215, "pattern (all files)"="*.config", "pattern label"="Configuración SEC") -> ("selected path"=w210:path, "cancelled"=w217:bool, "error out"=w213:errorcluster)  [unwired: 9 in, 1 out]
        n110 = call <vilib>:"Clear Errors.vi"("error in (no error)"=w213) -> ()  [unwired: 5 in, 2 out]
        n111 = case shown="False" w217 {
          tunnel: w210 -> [w236 _]
          tunnel: w209 -> [w223 w254]
          tunnel: [w222 w254] -> w206
          tunnel: w208 -> [_ _]
          tunnel: w207 -> [w220 w253]
          tunnel: [w219 w253] -> w205
          tunnel: [w224 w252] -> w204
          tunnel: w203 -> [_ w252]
          frame False {
            n112 = Open/Create/Replace File(file path (use dialog)=w236, operation (0:open)=T18."open", access (0:read/write)=enum16{"read/write", "read-only", "write-only"}."read-only") -> (refnum out=w234:refnum<file>, error out=w232:errorcluster)  [unwired: 3 in, 1 out]
            n113 = Read from Binary File(5:"", 8:w232, 11:w234) -> (0:w231:errorcluster, 2:w229:string, 3:w233:refnum<file>)  [unwired: 3 in, 1 out]
            n114 = Bundle(w223) -> (w228:T21)  [unwired: 1 in]
            n115 = Unflatten From String(type=w228, binary string=w229) -> (value=w227:T21)  [unwired: 3 in, 2 out]
            n116 = Close File(refnum=w233, error in=w231) -> (error out=w230:errorcluster)  [unwired: 1 out]
            n117 = Unbundle(w227) -> (w222:T17)
            n118 = call <vilib>:"Clear Errors.vi"("error in (no error)"=w230) -> ()  [unwired: 5 in, 2 out]
            n119 = for {
              tunnel: w222 -> [w251] mode=indexing
              tunnel: [w239] -> w224 mode=indexing
              n120 = Unbundle By Name(w251) -> ("Progs Data"=w238:variant)
              n121 = Variant To Data(type=cluster{"I/O Map":T19, "Prog":T20} {"I/O Map"={"Inputs"=[], "Outputs"=[]}, "Prog"={"Prog. Data"={"Tipo de Programa"="", "Operación"=0, "Pieza"=0, "Descripción"="", "Nombre Programa"="", "Autor"="", "Cód. Prog."=0, "Diseño"="", "Total Meds.:"=0, "Total Meds. Aux.:"=0}, "All Sequences"={"Measurement"={"STEPs"=[], "Main Error&Alarm"={"Main Error"={"RPN "=[], "Variables"=[], "Ctes"=[], "Formula"="", "Message"=""}, "Main Alarm 1"={"RPN "=[], "Variables"=[], "Ctes"=[], "Formula"="", "Message"=""}, "Main Alarm 2"={"RPN "=[], "Variables"=[], "Ctes"=[], "Formula"="", "Message"=""}, "Main Alarm 3"={"RPN "=[], "Variables"=[], "Ctes"=[], "Formula"="", "Message"=""}, "Main Alarm 4"={"RPN "=[], "Variables"=[], "Ctes"=[], "Formula"="", "Message"=""}}, "STEP Type"=refnum}, "AutoZero"={"STEPs"=[], "Main Error&Alarm"={"Main Error"={"RPN "=[], "Variables"=[], "Ctes"=[], "Formula"="", "Message"=""}, "Main Alarm 1"={"RPN "=[], "Variables"=[], "Ctes"=[], "Formula"="", "Message"=""}, "Main Alarm 2"={"RPN "=[], "Variables"=[], "Ctes"=[], "Formula"="", "Message"=""}, "Main Alarm 3"={"RPN "=[], "Variables"=[], "Ctes"=[], "Formula"="", "Message"=""}, "Main Alarm 4"={"RPN "=[], "Variables"=[], "Ctes"=[], "Formula"="", "Message"=""}}, "STEP Type"=refnum}, "Special"={"STEPs"=[], "Main Error&Alarm"={"Main Error"={"RPN "=[], "Variables"=[], "Ctes"=[], "Formula"="", "Message"=""}, "Main Alarm 1"={"RPN "=[], "Variables"=[], "Ctes"=[], "Formula"="", "Message"=""}, "Main Alarm 2"={"RPN "=[], "Variables"=[], "Ctes"=[], "Formula"="", "Message"=""}, "Main Alarm 3"={"RPN "=[], "Variables"=[], "Ctes"=[], "Formula"="", "Message"=""}, "Main Alarm 4"={"RPN "=[], "Variables"=[], "Ctes"=[], "Formula"="", "Message"=""}}, "STEP Type"=refnum}}}}, Variant=w238) -> (data=w241:cluster{"I/O Map":T19, "Prog":T20})  [unwired: 1 in, 1 out]
              n122 = Unbundle By Name(w241) -> ("Prog.Prog. Data.Cód. Prog."=w242:i32, "Prog.Prog. Data.Nombre Programa"=w244:string, "Prog.Prog. Data.Descripción"=w245:string, "Prog.Prog. Data.Pieza"=w246:i32, "Prog.Prog. Data.Diseño"=w248:string, "Prog.Prog. Data.Operación"=w249:i32, "Prog.Prog. Data.Tipo de Programa"=w240:string)
              n123 = Number To Decimal String(number=w242) -> (decimal integer string=w243:string)  [unwired: 1 in]
              n124 = Number To Decimal String(number=w246) -> (decimal integer string=w247:string)  [unwired: 1 in]
              n125 = Number To Decimal String(number=w249) -> (decimal integer string=w250:string)  [unwired: 1 in]
              n126 = Build Array(w243, w244, w245, w247, w248, w250, w240) -> (w239:string[])
            }
            n127 = property on="Editor de Programas" class="MCListbox (strict)"(error in=w220, "Val(Sgnl)"=0 ("Value (Signaling)")) -> (error out=w219:errorcluster)  [unwired: 1 in, 1 out]
          }
          frame True {
          }
        }
      }
      event "Save Cfg": Value Change {
        n128 = event-data() -> ()  [unwired: 1 in, 6 out]
        n129 = call <vilib>:"Application Directory.vi"() -> ("Application Directory"=w264:path)
        n130 = Build Path(base path=w264, name or relative path="Configuraciones") -> (appended path=w266:path)
        n131 = Bundle(w258) -> (w267:T21)  [unwired: 1 in]
        n132 = call "File Dialog2"("start path"=w266, "pattern (all files)"="*.config", "pattern label"="Configuración SEC") -> ("selected path"=w259:path, "cancelled"=w262:bool, "error out"=w263:errorcluster)  [unwired: 9 in, 1 out]
        n133 = Flatten To String(anything=w267, error in (no error)=w256) -> (data string=w268:string, error out=w255:errorcluster)  [unwired: 2 in, 1 out]
        n134 = call <vilib>:"Clear Errors.vi"("error in (no error)"=w263) -> ()  [unwired: 5 in, 2 out]
        n135 = case shown="False" w262 {
          tunnel: w268 -> [w276 _]
          tunnel: w259 -> [w272 _]
          frame False {
            n136 = Open/Create/Replace File(file path (use dialog)=w272, operation (0:open)=T18."open or create", access (0:read/write)=enum16{"read/write", "read-only", "write-only"}."write-only") -> (refnum out=w273:refnum<file>, error out=w270:errorcluster)  [unwired: 3 in, 1 out]
            n137 = Write to Binary File(file (use dialog)=w273, data=w276, error in=w270) -> (refnum out=w271:refnum<file>, error out=w269:errorcluster)  [unwired: 3 in, 1 out]
            n138 = Close File(refnum=w271, error in=w269) -> ()  [unwired: 2 out]
          }
          frame True {
          }
        }
      }
      event "New Prog": Value Change {
        w287 = T12 {"File Direction"=path "", "Progs Data"=variant}  # Progs
        n139 = event-data() -> ()  [unwired: 1 in, 1 out]
        n140 = Matrix Size(0:w307) -> (1:w290:i32)  [unwired: 1 out]
        n141 = Number To Decimal String(number=w290) -> (decimal integer string=w298:string)  [unwired: 1 in]
        n142 = Index Array(array=w279, index=w278) -> (element=w277:T12)
        n143 = call "Config Program Type vi.vi"("error in (no error)"=w286, "SEQ"=w284) -> ("error out"=w285:errorcluster, "Program Type"=w280:string, "SEQ Out"=w283:refnum<queue>)  [unwired: 7 in]
        n144 = Concatenate Strings("Cod. Prog. ", w298) -> (w304:string)
        n145 = Concatenate Strings("Nombre Programa ", w298) -> (w303:string)
        n146 = Concatenate Strings("Descripción ", w298) -> (w302:string)
        n147 = Concatenate Strings("Pieza ", w298) -> (w301:string)
        n148 = Concatenate Strings("Diseño ", w298) -> (w300:string)
        n149 = Concatenate Strings("Operación ", w298) -> (w299:string)
        n150 = Build Array(w304, w303, w302, w301, w300, w299, w280) -> (w305:string[])
        n151 = Bundle("Progs"=w277, "Program Type"=w280) -> (w281:T22)  [unwired: 1 in]
        n152 = To Variant(anything=w281) -> (Variant=w282:variant)
        n153 = call-poly "Enqueue Message.vi"("error in (no error)"=w285, "Message Data"=w282, "Message"="INIT", "Message Queue"=w283) -> ("error out"=w288:errorcluster)  [unwired: 6 in, 1 out]
        n154 = Insert Into Array(array=w279, index=w290, new element=w287) -> (w291:T17)
        n155 = Insert Into Array(array=w307, index (row)=w290, new element=w305) -> (w308:string[][])  [unwired: 1 in]
        n156 = property on="Editor de Programas" class="MCListbox (strict)"(error in=w288, "Value"=w290) -> (error out=w306:errorcluster)  [unwired: 1 in, 1 out]
      }
      event "HOME": Value Change {
        n157 = event-data() -> ()  [unwired: 1 in, 1 out]
        n158 = property on="Tab Control 2" class="TabCtl (strict)"(error in=w311, "Value"=enum32{"HOME", "PIC", "TAB"}."HOME" ("Tab Control 2")) -> (error out=w315:errorcluster)  [unwired: 1 in, 1 out]
        n159 = property on="Tab Control" class="TabCtl (strict)"(error in=w311, "Value"=enum32{"HOME", "SEC", "MIMIC", "MESSAGE"}."HOME" ("Tab Control")) -> (error out=w329:errorcluster)  [unwired: 1 in, 1 out]
        n160 = property on="SEC" class="Bool (strict)"(error in=w311, "Value"=FALSE ("CICLO")) -> (error out=w331:errorcluster)  [unwired: 1 in, 1 out]
        n161 = property on="MIMIC" class="Bool (strict)"(error in=w311, "Value"=FALSE ("CONFIG.")) -> (error out=w318:errorcluster)  [unwired: 1 in, 1 out]
        n162 = property on="MESSAGE" class="Bool (strict)"(error in=w311, "Value"=FALSE ("CONFIG.")) -> (error out=w309:errorcluster)  [unwired: 1 in, 1 out]
        n163 = property on="MESSAGE" class="Bool (strict)"(error in=w311, "DisabledEnum"=T7."Enabled" ("Disabled")) -> (error out=w314:errorcluster)  [unwired: 1 in, 1 out]
        n164 = property on="SEC" class="Bool (strict)"(error in=w311, "DisabledEnum"=T7."Enabled" ("Disabled")) -> (error out=w319:errorcluster)  [unwired: 1 in, 1 out]
        n165 = property on="MIMIC" class="Bool (strict)"(error in=w311, "DisabledEnum"=T7."Enabled" ("Disabled")) -> (error out=w320:errorcluster)  [unwired: 1 in, 1 out]
        n166 = property on="HOME" class="Bool (strict)"(error in=w311, "DisabledEnum"=T7."Disabled" ("Disabled")) -> (error out=w310:errorcluster)  [unwired: 1 in, 1 out]
        n167 = Merge Errors(w315, w314, w319, w320, w329, w331, w318, w309, w310) -> (w327:errorcluster)
      }
      event "SEC": Value Change {
        w332 = T3 {"Boolean 36"=FALSE, "Boolean 3"=FALSE, "Boolean 35"=FALSE, "Boolean 34"=FALSE, "Boolean 33"=FALSE, "Boolean 32"=FALSE, "Boolean 16"=FALSE, "Boolean 17"=FALSE, "Boolean 26"=FALSE, "Boolean 25"=FALSE, "Boolean 24"=FALSE, "Boolean 23"=FALSE, "Boolean 37"=FALSE, "Boolean 1"=FALSE, "Boolean 15"=FALSE, "Boolean 4"=FALSE, "Boolean 5"=FALSE, "Boolean 6"=FALSE, "Boolean 7"=FALSE, "Boolean 8"=FALSE, "Boolean 9"=FALSE, "Boolean 10"=FALSE, "Boolean 11"=FALSE, "Boolean 12"=FALSE, "Boolean 38"=FALSE, "Boolean 21"=FALSE, "Boolean 22"=FALSE, "Boolean 20"=FALSE, "Boolean 19"=FALSE, "Boolean 18"=FALSE, "Boolean 40"=FALSE, "Boolean 39"=FALSE} ("View Out")
        n168 = event-data() -> ()  [unwired: 1 in, 1 out]
        n169 = Index Array(array=w339, index (row)=w338, index (col)=6) -> (element=w336:string)
        n170 = case shown="Default" w336 {
          tunnel: [T7."Enabled" ("Disabled") T7."Disabled and Grayed Out" ("Disabled")] -> w335
          frame Default {
          }
          frame "CAP" {
          }
        }
        n171 = property on="Start Sec Special" class="Bool"(error in=w334, "DisabledEnum"=w335) -> (error out=w333:errorcluster)  [unwired: 1 in, 1 out]
        n172 = property on="Tab Control 2" class="TabCtl (strict)"(error in=w334, "Value"=enum32{"HOME", "PIC", "TAB"}."PIC" ("Tab Control 2")) -> (error out=w348:errorcluster)  [unwired: 1 in, 1 out]
        n173 = property on="Tab Control" class="TabCtl (strict)"(error in=w334, "Value"=enum32{"HOME", "SEC", "MIMIC", "MESSAGE"}."SEC" ("Tab Control")) -> (error out=w357:errorcluster)  [unwired: 1 in, 1 out]
        n174 = property on="MESSAGE" class="Bool (strict)"(error in=w334, "Value"=FALSE ("CICLO")) -> (error out=w340:errorcluster)  [unwired: 1 in, 1 out]
        n175 = property on="HOME" class="Bool (strict)"(error in=w334, "Value"=FALSE ("CICLO")) -> (error out=w341:errorcluster)  [unwired: 1 in, 1 out]
        n176 = property on="MIMIC" class="Bool (strict)"(error in=w334, "Value"=FALSE ("CONFIG.")) -> (error out=w342:errorcluster)  [unwired: 1 in, 1 out]
        n177 = property on="HOME" class="Bool (strict)"(error in=w334, "DisabledEnum"=T7."Enabled" ("Disabled")) -> (error out=w347:errorcluster)  [unwired: 1 in, 1 out]
        n178 = property on="MIMIC" class="Bool (strict)"(error in=w334, "DisabledEnum"=T7."Enabled" ("Disabled")) -> (error out=w346:errorcluster)  [unwired: 1 in, 1 out]
        n179 = property on="MESSAGE" class="Bool (strict)"(error in=w334, "DisabledEnum"=T7."Enabled" ("Disabled")) -> (error out=w345:errorcluster)  [unwired: 1 in, 1 out]
        n180 = property on="SEC" class="Bool (strict)"(error in=w334, "DisabledEnum"=T7."Disabled" ("Disabled")) -> (error out=w343:errorcluster)  [unwired: 1 in, 1 out]
        n181 = Merge Errors(w333, w348, w347, w346, w345, w357, w340, w341, w342, w343) -> (w359:errorcluster)
        n182 = global write "DO Monitoring Global Variables.vi" "View Out"(w332) -> ()
        n183 = global write "DO Monitoring Global Variables.vi" "View Out 2"(w332) -> ()
        n184 = global write "DO Monitoring Global Variables.vi" "View Out 3"(w332) -> ()
        n185 = global write "DO Monitoring Global Variables.vi" "View Out 4"(w332) -> ()
        n186 = global write "DO Monitoring Global Variables.vi" "View Out 5"(w332) -> ()
      }
      event "MIMIC": Value Change {
        n187 = event-data() -> ()  [unwired: 1 in, 1 out]
        n188 = property on="Tab Control 2" class="TabCtl (strict)"(error in=w362, "Value"=enum32{"HOME", "PIC", "TAB"}."TAB" ("Tab Control 2")) -> (error out=w367:errorcluster)  [unwired: 1 in, 1 out]
        n189 = property on="Tab Control" class="TabCtl (strict)"(error in=w362, "Value"=enum32{"HOME", "SEC", "MIMIC", "MESSAGE"}."MIMIC" ("Tab Control")) -> (error out=w382:errorcluster)  [unwired: 1 in, 1 out]
        n190 = property on="HOME" class="Bool (strict)"(error in=w362, "Value"=FALSE ("CICLO")) -> (error out=w384:errorcluster)  [unwired: 1 in, 1 out]
        n191 = property on="SEC" class="Bool (strict)"(error in=w362, "Value"=FALSE ("CONFIG.")) -> (error out=w372:errorcluster)  [unwired: 1 in, 1 out]
        n192 = property on="MESSAGE" class="Bool (strict)"(error in=w362, "Value"=FALSE ("CONFIG.")) -> (error out=w363:errorcluster)  [unwired: 1 in, 1 out]
        n193 = property on="MESSAGE" class="Bool (strict)"(error in=w362, "DisabledEnum"=T7."Enabled" ("Disabled")) -> (error out=w366:errorcluster)  [unwired: 1 in, 1 out]
        n194 = property on="HOME" class="Bool (strict)"(error in=w362, "DisabledEnum"=T7."Enabled" ("Disabled")) -> (error out=w373:errorcluster)  [unwired: 1 in, 1 out]
        n195 = property on="SEC" class="Bool (strict)"(error in=w362, "DisabledEnum"=T7."Enabled" ("Disabled")) -> (error out=w374:errorcluster)  [unwired: 1 in, 1 out]
        n196 = property on="MIMIC" class="Bool (strict)"(error in=w362, "DisabledEnum"=T7."Disabled" ("Disabled")) -> (error out=w364:errorcluster)  [unwired: 1 in, 1 out]
        n197 = Merge Errors(w367, w366, w373, w374, w382, w384, w372, w363, w364) -> (w381:errorcluster)
      }
      event "MESSAGE": Value Change {
        n198 = event-data() -> ()  [unwired: 1 in, 1 out]
        n199 = property on="Tab Control 2" class="TabCtl (strict)"(error in=w387, "Value"=enum32{"HOME", "PIC", "TAB"}."TAB" ("Tab Control 2")) -> (error out=w390:errorcluster)  [unwired: 1 in, 1 out]
        n200 = property on="Tab Control" class="TabCtl (strict)"(error in=w387, "Value"=enum32{"HOME", "SEC", "MIMIC", "MESSAGE"}."MESSAGE" ("Tab Control")) -> (error out=w402:errorcluster)  [unwired: 1 in, 1 out]
        n201 = property on="HOME" class="Bool (strict)"(error in=w387, "Value"=FALSE ("CICLO")) -> (error out=w404:errorcluster)  [unwired: 1 in, 1 out]
        n202 = property on="SEC" class="Bool (strict)"(error in=w387, "Value"=FALSE ("CONFIG.")) -> (error out=w396:errorcluster)  [unwired: 1 in, 1 out]
        n203 = property on="MIMIC" class="Bool (strict)"(error in=w387, "Value"=FALSE ("CONFIG.")) -> (error out=w385:errorcluster)  [unwired: 1 in, 1 out]
        n204 = property on="MIMIC" class="Bool (strict)"(error in=w387, "DisabledEnum"=T7."Enabled" ("Disabled")) -> (error out=w389:errorcluster)  [unwired: 1 in, 1 out]
        n205 = property on="HOME" class="Bool (strict)"(error in=w387, "DisabledEnum"=T7."Enabled" ("Disabled")) -> (error out=w397:errorcluster)  [unwired: 1 in, 1 out]
        n206 = property on="SEC" class="Bool (strict)"(error in=w387, "DisabledEnum"=T7."Enabled" ("Disabled")) -> (error out=w398:errorcluster)  [unwired: 1 in, 1 out]
        n207 = property on="MESSAGE" class="Bool (strict)"(error in=w387, "DisabledEnum"=T7."Disabled" ("Disabled")) -> (error out=w386:errorcluster)  [unwired: 1 in, 1 out]
        n208 = Merge Errors(w390, w389, w397, w398, w402, w404, w396, w385, w386) -> (w394:errorcluster)
      }
      event "I/O Config": Value Change {
        n209 = event-data() -> ()  [unwired: 1 in, 1 out]
        n210 = call-poly "Enqueue Message.vi"("error in (no error)"=w409, "Message"="Config:IO", "Message Queue"=w410) -> ("error out"=w408:errorcluster, "dup Message Queue"=w413:refnum<queue>)  [unwired: 7 in]
        n211 = call-poly "Enqueue Message.vi"("error in (no error)"=w408, "Message"="Config:Get", "Message Queue"=w413) -> ("error out"=w407:errorcluster)  [unwired: 7 in, 1 out]
      }
      event "Config Prog": Value Change {
        n212 = event-data() -> ()  [unwired: 1 in, 1 out]
        n213 = Index Array(array=w421, index (row)=w420, index (col)=6 ("disabled index (col)")) -> (element=w418:string)
        n214 = To Variant(anything=w418) -> (Variant=w417:variant)
        n215 = call-poly "Enqueue Message.vi"("error in (no error)"=w424, "Message Data"=w417, "Message"="Config", "Message Queue"=w423) -> ("error out"=w425:errorcluster, "dup Message Queue"=w426:refnum<queue>)  [unwired: 6 in]
        n216 = call-poly "Enqueue Message.vi"("Message"="Config:Get", "Message Queue"=w426) -> ()  [unwired: 8 in, 2 out]
      }
      event User Event {
        n217 = event-data() -> ("Config Data"=w431:variant)  [unwired: 1 in]
        n218 = in-place {
          in-place-border: w431 -> [w450]
          n219 = in-place-array #1(w449, w442) -> (w452:T12)
          n220 = Bundle By Name(cluster=w452, "Progs Data"=w450) -> (w451:T12)
          n221 = in-place-array #1(w451) -> (w448:T17)  [unwired: 1 out]
        }
        n222 = Variant To Data(error in=w430, type=cluster{"I/O Map":T19, "Prog":T20} {"I/O Map"={"Inputs"=[], "Outputs"=[]}, "Prog"={"Prog. Data"={"Tipo de Programa"="", "Operación"=0, "Pieza"=0, "Descripción"="", "Nombre Programa"="", "Autor"="", "Cód. Prog."=0, "Diseño"="", "Total Meds.:"=0, "Total Meds. Aux.:"=0}, "All Sequences"={"Measurement"={"STEPs"=[], "Main Error&Alarm"={"Main Error"={"RPN "=[], "Variables"=[], "Ctes"=[], "Formula"="", "Message"=""}, "Main Alarm 1"={"RPN "=[], "Variables"=[], "Ctes"=[], "Formula"="", "Message"=""}, "Main Alarm 2"={"RPN "=[], "Variables"=[], "Ctes"=[], "Formula"="", "Message"=""}, "Main Alarm 3"={"RPN "=[], "Variables"=[], "Ctes"=[], "Formula"="", "Message"=""}, "Main Alarm 4"={"RPN "=[], "Variables"=[], "Ctes"=[], "Formula"="", "Message"=""}}, "STEP Type"=refnum}, "AutoZero"={"STEPs"=[], "Main Error&Alarm"={"Main Error"={"RPN "=[], "Variables"=[], "Ctes"=[], "Formula"="", "Message"=""}, "Main Alarm 1"={"RPN "=[], "Variables"=[], "Ctes"=[], "Formula"="", "Message"=""}, "Main Alarm 2"={"RPN "=[], "Variables"=[], "Ctes"=[], "Formula"="", "Message"=""}, "Main Alarm 3"={"RPN "=[], "Variables"=[], "Ctes"=[], "Formula"="", "Message"=""}, "Main Alarm 4"={"RPN "=[], "Variables"=[], "Ctes"=[], "Formula"="", "Message"=""}}, "STEP Type"=refnum}, "Special"={"STEPs"=[], "Main Error&Alarm"={"Main Error"={"RPN "=[], "Variables"=[], "Ctes"=[], "Formula"="", "Message"=""}, "Main Alarm 1"={"RPN "=[], "Variables"=[], "Ctes"=[], "Formula"="", "Message"=""}, "Main Alarm 2"={"RPN "=[], "Variables"=[], "Ctes"=[], "Formula"="", "Message"=""}, "Main Alarm 3"={"RPN "=[], "Variables"=[], "Ctes"=[], "Formula"="", "Message"=""}, "Main Alarm 4"={"RPN "=[], "Variables"=[], "Ctes"=[], "Formula"="", "Message"=""}}, "STEP Type"=refnum}}}}, Variant=w431) -> (data=w446:cluster{"I/O Map":T19, "Prog":T20}, error out=w447:errorcluster)
        n223 = Unbundle By Name(w446) -> ("Prog.Prog. Data.Cód. Prog."=w441:i32, "Prog.Prog. Data.Nombre Programa"=w439:string, "Prog.Prog. Data.Descripción"=w438:string, "Prog.Prog. Data.Pieza"=w437:i32, "Prog.Prog. Data.Diseño"=w435:string, "Prog.Prog. Data.Operación"=w434:i32, "Prog.Prog. Data.Tipo de Programa"=w432:string)
        n224 = Number To Decimal String(number=w441) -> (decimal integer string=w440:string)  [unwired: 1 in]
        n225 = Number To Decimal String(number=w437) -> (decimal integer string=w436:string)  [unwired: 1 in]
        n226 = Number To Decimal String(number=w434) -> (decimal integer string=w433:string)  [unwired: 1 in]
        n227 = Build Array(w440, w439, w438, w436, w435, w433, w432) -> (w443:string[])
        n228 = Replace Array Subset(array=w445, new element=w443, index (row)=w442) -> (w444:string[][])  [unwired: 1 in]
      }
      event "Start Sec A-Z": Value Change {
        w454 = T3 {"Boolean 36"=FALSE, "Boolean 3"=FALSE, "Boolean 35"=FALSE, "Boolean 34"=FALSE, "Boolean 33"=FALSE, "Boolean 32"=FALSE, "Boolean 16"=FALSE, "Boolean 17"=FALSE, "Boolean 26"=FALSE, "Boolean 25"=FALSE, "Boolean 24"=FALSE, "Boolean 23"=FALSE, "Boolean 37"=FALSE, "Boolean 1"=FALSE, "Boolean 15"=FALSE, "Boolean 4"=FALSE, "Boolean 5"=FALSE, "Boolean 6"=FALSE, "Boolean 7"=FALSE, "Boolean 8"=FALSE, "Boolean 9"=FALSE, "Boolean 10"=FALSE, "Boolean 11"=FALSE, "Boolean 12"=FALSE, "Boolean 38"=FALSE, "Boolean 21"=FALSE, "Boolean 22"=FALSE, "Boolean 20"=FALSE, "Boolean 19"=FALSE, "Boolean 18"=FALSE, "Boolean 40"=FALSE, "Boolean 39"=FALSE} ("View Out")
        w461 = T13 {"Row"=-2, "Column"=-2} ("Active Cell:Active Cell")
        w464 = T13 {"Row"=0, "Column"=-2} ("Active Cell:Active Cell")
        w465 = u32 4110335
        w462 = u32 16448250
        n229 = event-data() -> ()  [unwired: 1 in, 1 out]
        n230 = To Variant(anything="Auto-Zero") -> (Variant=w467:variant)
        n231 = call-poly "Enqueue Message.vi"("error in (no error)"=w457, "Message Data"=w467, "Message"="Start", "Message Queue"=w474) -> ("error out"=w463:errorcluster)  [unwired: 6 in, 1 out]
        n232 = call-poly "Enqueue Message.vi"("error in (no error)"=w457, "Message"="Init", "Message Queue"=w456) -> ()  [unwired: 7 in, 2 out]
        n233 = property on="Acept" class="Bool"("Val(Sgnl)"=FALSE) -> ()  [unwired: 2 in, 2 out]
        n234 = property on="Cond. Avan." class="Tbl (strict)"(error in=w463, "Active Cell"=w461, "Cell BG Color"=w462) -> (error out=w466:errorcluster)  [unwired: 1 in, 1 out]
        n235 = property on="Current Sequence" class="Tbl (strict)"(error in=w463, "Active Cell"=w461, "Cell BG Color"=w462) -> (error out=w469:errorcluster)  [unwired: 1 in, 1 out]
        n236 = global write "DO Monitoring Global Variables.vi" "View Out"(w454) -> ()
        n237 = global write "DO Monitoring Global Variables.vi" "View Out 2"(w454) -> ()
        n238 = global write "DO Monitoring Global Variables.vi" "View Out 3"(w454) -> ()
        n239 = global write "DO Monitoring Global Variables.vi" "View Out 4"(w454) -> ()
        n240 = global write "DO Monitoring Global Variables.vi" "View Out 5"(w454) -> ()
        n241 = property on="Cond. Avan." class="Tbl (strict)"(error in=w466, "Active Cell"=w464, "Cell BG Color"=w465) -> (error out=w460:errorcluster)  [unwired: 1 in, 1 out]
        n242 = property on="Current Sequence" class="Tbl (strict)"(error in=w469, "Active Cell"=w464, "Cell BG Color"=w465) -> (error out=w459:errorcluster)  [unwired: 1 in, 1 out]
        n243 = Merge Errors(w460, w459) -> (w455:errorcluster)
      }
      event "Start Sec Ciclo": Value Change {
        w476 = T3 {"Boolean 36"=FALSE, "Boolean 3"=FALSE, "Boolean 35"=FALSE, "Boolean 34"=FALSE, "Boolean 33"=FALSE, "Boolean 32"=FALSE, "Boolean 16"=FALSE, "Boolean 17"=FALSE, "Boolean 26"=FALSE, "Boolean 25"=FALSE, "Boolean 24"=FALSE, "Boolean 23"=FALSE, "Boolean 37"=FALSE, "Boolean 1"=FALSE, "Boolean 15"=FALSE, "Boolean 4"=FALSE, "Boolean 5"=FALSE, "Boolean 6"=FALSE, "Boolean 7"=FALSE, "Boolean 8"=FALSE, "Boolean 9"=FALSE, "Boolean 10"=FALSE, "Boolean 11"=FALSE, "Boolean 12"=FALSE, "Boolean 38"=FALSE, "Boolean 21"=FALSE, "Boolean 22"=FALSE, "Boolean 20"=FALSE, "Boolean 19"=FALSE, "Boolean 18"=FALSE, "Boolean 40"=FALSE, "Boolean 39"=FALSE} ("View Out")
        w483 = T13 {"Row"=0, "Column"=-2} ("Active Cell:Active Cell")
        w484 = u32 4110335
        w486 = T13 {"Row"=-2, "Column"=-2} ("Active Cell:Active Cell")
        w485 = u32 16448250
        n244 = event-data() -> ()  [unwired: 1 in, 1 out]
        n245 = To Variant(anything="Measurement") -> (Variant=w489:variant)
        n246 = call-poly "Enqueue Message.vi"("error in (no error)"=w479, "Message"="Init", "Message Queue"=w478) -> ()  [unwired: 7 in, 2 out]
        n247 = call-poly "Enqueue Message.vi"("error in (no error)"=w479, "Message Data"=w489, "Message"="Start", "Message Queue"=w495) -> ("error out"=w487:errorcluster)  [unwired: 6 in, 1 out]
        n248 = property on="Acept" class="Bool"("Val(Sgnl)"=FALSE) -> ()  [unwired: 2 in, 2 out]
        n249 = property on="Cond. Avan." class="Tbl (strict)"(error in=w487, "Active Cell"=w486, "Cell BG Color"=w485) -> (error out=w488:errorcluster)  [unwired: 1 in, 1 out]
        n250 = property on="Current Sequence" class="Tbl (strict)"(error in=w487, "Active Cell"=w486, "Cell BG Color"=w485) -> (error out=w491:errorcluster)  [unwired: 1 in, 1 out]
        n251 = property on="Cond. Avan." class="Tbl (strict)"(error in=w488, "Active Cell"=w483, "Cell BG Color"=w484) -> (error out=w482:errorcluster)  [unwired: 1 in, 1 out]
        n252 = property on="Current Sequence" class="Tbl (strict)"(error in=w491, "Active Cell"=w483, "Cell BG Color"=w484) -> (error out=w481:errorcluster)  [unwired: 1 in, 1 out]
        n253 = Merge Errors(w482, w481) -> (w477:errorcluster)
        n254 = global write "DO Monitoring Global Variables.vi" "View Out"(w476) -> ()
        n255 = global write "DO Monitoring Global Variables.vi" "View Out 2"(w476) -> ()
        n256 = global write "DO Monitoring Global Variables.vi" "View Out 3"(w476) -> ()
        n257 = global write "DO Monitoring Global Variables.vi" "View Out 4"(w476) -> ()
        n258 = global write "DO Monitoring Global Variables.vi" "View Out 5"(w476) -> ()
      }
      event "Start Sec Special": Value Change {
        w498 = T3 {"Boolean 36"=FALSE, "Boolean 3"=FALSE, "Boolean 35"=FALSE, "Boolean 34"=FALSE, "Boolean 33"=FALSE, "Boolean 32"=FALSE, "Boolean 16"=FALSE, "Boolean 17"=FALSE, "Boolean 26"=FALSE, "Boolean 25"=FALSE, "Boolean 24"=FALSE, "Boolean 23"=FALSE, "Boolean 37"=FALSE, "Boolean 1"=FALSE, "Boolean 15"=FALSE, "Boolean 4"=FALSE, "Boolean 5"=FALSE, "Boolean 6"=FALSE, "Boolean 7"=FALSE, "Boolean 8"=FALSE, "Boolean 9"=FALSE, "Boolean 10"=FALSE, "Boolean 11"=FALSE, "Boolean 12"=FALSE, "Boolean 38"=FALSE, "Boolean 21"=FALSE, "Boolean 22"=FALSE, "Boolean 20"=FALSE, "Boolean 19"=FALSE, "Boolean 18"=FALSE, "Boolean 40"=FALSE, "Boolean 39"=FALSE} ("View Out")
        w505 = T13 {"Row"=0, "Column"=-2} ("Active Cell:Active Cell")
        w506 = u32 4110335
        w508 = T13 {"Row"=-2, "Column"=-2} ("Active Cell:Active Cell")
        w507 = u32 16448250
        n259 = event-data() -> ()  [unwired: 1 in, 1 out]
        n260 = To Variant(anything="Special") -> (Variant=w511:variant)
        n261 = call-poly "Enqueue Message.vi"("error in (no error)"=w501, "Message"="Init", "Message Queue"=w500) -> ()  [unwired: 7 in, 2 out]
        n262 = call-poly "Enqueue Message.vi"("error in (no error)"=w501, "Message Data"=w511, "Message"="Start", "Message Queue"=w517) -> ("error out"=w509:errorcluster)  [unwired: 6 in, 1 out]
        n263 = property on="Cond. Avan." class="Tbl (strict)"(error in=w509, "Active Cell"=w508, "Cell BG Color"=w507) -> (error out=w510:errorcluster)  [unwired: 1 in, 1 out]
        n264 = property on="Current Sequence" class="Tbl (strict)"(error in=w509, "Active Cell"=w508, "Cell BG Color"=w507) -> (error out=w513:errorcluster)  [unwired: 1 in, 1 out]
        n265 = property on="Acept" class="Bool"("Val(Sgnl)"=FALSE) -> ()  [unwired: 2 in, 2 out]
        n266 = property on="Cond. Avan." class="Tbl (strict)"(error in=w510, "Active Cell"=w505, "Cell BG Color"=w506) -> (error out=w504:errorcluster)  [unwired: 1 in, 1 out]
        n267 = property on="Current Sequence" class="Tbl (strict)"(error in=w513, "Active Cell"=w505, "Cell BG Color"=w506) -> (error out=w503:errorcluster)  [unwired: 1 in, 1 out]
        n268 = Merge Errors(w504, w503) -> (w499:errorcluster)
        n269 = global write "DO Monitoring Global Variables.vi" "View Out"(w498) -> ()
        n270 = global write "DO Monitoring Global Variables.vi" "View Out 2"(w498) -> ()
        n271 = global write "DO Monitoring Global Variables.vi" "View Out 3"(w498) -> ()
        n272 = global write "DO Monitoring Global Variables.vi" "View Out 4"(w498) -> ()
        n273 = global write "DO Monitoring Global Variables.vi" "View Out 5"(w498) -> ()
      }
      event "Acept": Value Change {
        n274 = event-data() -> ()  [unwired: 1 in, 1 out]
        n275 = flat-sequence {
          tunnel: [w526] -> w523
          tunnel: w522 -> [w526]
          tunnel: w523 -> [w529]
          tunnel: [w528] -> w521
          tunnel: w521 -> [w548]
          tunnel: [w547] -> w520
          frame #0 {
            n276 = local write "Acept"(FALSE ("Acept")) -> ()
          }
          frame #1 {
            n277 = for {
              N: 13 -> [_]
              shift-right: [w537] -> _
              shift-left: "" ("Boolean Text.Text") -> [w542]
              tunnel: w529 -> [w534]
              tunnel: [w533] -> w528
              i -> [w546]
              n278 = Equal?(x=0, y=w546) -> (x = y?=w544:bool)
              n279 = Select(t="CONTROLANDO" ("Boolean Text.Text"), s=w544, f=". " ("Boolean Text.Text")) -> (s? t:f=w541:string)
              n280 = Concatenate Strings(w542, w541) -> (w538:string)
              n281 = Equal?(x="CONTROLANDO. . . " ("Boolean Text.Text"), y=w538) -> (x = y?=w539:bool)
              n282 = property on="Acept" class="Bool"(error in=w534, "BoolText.Text"=w538) -> (error out=w533:errorcluster)  [unwired: 1 in, 1 out]
              n283 = Select(t="CONTROLANDO" ("Boolean Text.Text"), s=w539, f=w538) -> (s? t:f=w537:string)
              n284 = Wait (ms)(milliseconds to wait=u32 200) -> ()  [unwired: 1 out]
            }
          }
          frame #2 {
            n285 = property on="Acept" class="Bool"(error in=w548, "BoolText.Text"="       ACEPTADO" ("Boolean Text.Text")) -> (error out=w547:errorcluster)  [unwired: 1 in, 1 out]
            "Acept" <- TRUE ("Acept")
          }
        }
      }
      event "Conf In", "Conf In 2", "Conf In 3", "Conf In 4", "Conf In 5", "Angle": Value Change {
        w568 = T23 {"Encoder"=0.0, "DI"=[], "DO"=[]} ("Control Data")
        n286 = event-data() -> ()  [unwired: 1 in, 1 out]
        n287 = Unbundle By Name(w556) -> ("CTRL HWSync1"=w551:refnum<notifier>, "CTRL HWSync2"=w552:refnum<notifier>, "CTRL HWSync3"=w553:refnum<notifier>, "CTRL HWSync4"=w554:refnum<notifier>, "CTRL HWSync5"=w555:refnum<notifier>)
        n288 = Cluster To Array(cluster="Conf In") -> (array=w577:bool[])
        n289 = Cluster To Array(cluster="Conf In 2") -> (array=w576:bool[])
        n290 = Cluster To Array(cluster="Conf In 3") -> (array=w570:bool[])
        n291 = Cluster To Array(cluster="Conf In 4") -> (array=w569:bool[])
        n292 = Cluster To Array(cluster="Conf In 5") -> (array=w573:bool[])
        n293 = Bundle By Name(cluster=w568, "DI"=w577, "Encoder"="Angle") -> (w580:T23)
        n294 = Bundle By Name(cluster=w568, "DI"=w576) -> (w574:T23)
        n295 = Bundle By Name(cluster=w568, "DI"=w570) -> (w565:T23)
        n296 = Bundle By Name(cluster=w568, "DI"=w569) -> (w564:T23)
        n297 = Bundle By Name(cluster=w568, "DI"=w573) -> (w571:T23)
        n298 = call "Send CTRL Notification.vi"("error in (no error)"=w563, "Control Data"=w580, "CTRL Data Notifier in"=w551) -> ("error out"=w562:errorcluster)  [unwired: 7 in, 1 out]
        n299 = call "Send CTRL Notification.vi"("error in (no error)"=w563, "Control Data"=w574, "CTRL Data Notifier in"=w552) -> ("error out"=w561:errorcluster)  [unwired: 7 in, 1 out]
        n300 = call "Send CTRL Notification.vi"("error in (no error)"=w563, "Control Data"=w565, "CTRL Data Notifier in"=w553) -> ("error out"=w560:errorcluster)  [unwired: 7 in, 1 out]
        n301 = call "Send CTRL Notification.vi"("error in (no error)"=w563, "Control Data"=w564, "CTRL Data Notifier in"=w554) -> ("error out"=w559:errorcluster)  [unwired: 7 in, 1 out]
        n302 = call "Send CTRL Notification.vi"("error in (no error)"=w563, "Control Data"=w571, "CTRL Data Notifier in"=w555) -> ("error out"=w558:errorcluster)  [unwired: 7 in, 1 out]
        n303 = Merge Errors(w562, w561, w560, w559, w558) -> (w557:errorcluster)
      }
      event Panel Close? {
        n304 = event-data() -> ()  [unwired: 1 in, 1 out]
        n305 = call-poly "Enqueue Message.vi"("error in (no error)"=w591, "Message"="EXIT", "Message Queue"=w587) -> ("error out"=w590:errorcluster)  [unwired: 7 in, 1 out]
        n306 = call-poly "Enqueue Message.vi"("error in (no error)"=w590, "Message"="EXIT", "Message Queue"=w588) -> ("error out"=w589:errorcluster)  [unwired: 7 in, 1 out]
        n307 = event-data("Discard?"=TRUE) -> ()  [unwired: 1 in, 1 out]
      }
    }
    n308 = property on="Editor de Programas" class="MCListbox (strict)"(error in=w109, "ItemNames"=w103) -> ()  [unwired: 1 in, 2 out]
  }
  n309 = while {
    tunnel: [w604] -> _
    tunnel: w97 -> [w600]
    tunnel: w56 -> [w599]
    tunnel: w94 -> [w598]
    shift-right: [w596] -> _
    shift-left: T6 {"HWS1"="", "HWS2"="", "HWS3"="", "HWS4"="", "HWS5"="", "MATH"=""} -> [w597]
    stop <- w605 stop-if-true
    # "HAL Message Switch Loop"
    n310 = call "Dequeue Message.vi"("error in (no error)"=w599, "Message Queue"=w600) -> ("error out"=w603:errorcluster, "Message Data"=w602:variant, "Message"=w601:string)  [unwired: 6 in, 1 out]
    n311 = case shown="Default" w601 {
      selector: w601 -> [w612 _ _ _]
      tunnel: w603 -> [w616 w841 w844 w870]
      tunnel: w602 -> [w611 _ _ w872]
      tunnel: [_ TRUE _ _] -> w605
      tunnel: [w616 w841 w843 w869] -> w604
      tunnel: w598 -> [_ _ _ w871]
      tunnel: w597 -> [w609 w840 _ w868]
      tunnel: [w610 w840 T6 {"HWS1"="", "HWS2"="", "HWS3"="", "HWS4"="", "HWS5"="", "MATH"=""} w868] -> w596
      frame Default {
        n312 = Get Date/Time In Seconds() -> (seconds since 1Jan1904=w607:timestamp)
        n313 = Match Pattern(string=w612, regular expression=":") -> (before substring=w614:string, after substring=w613:string)  [unwired: 1 in, 2 out]
        n314 = Format Date/Time String(time format string (%c)="%H:%M:%S%3u ", seconds (now)=w607) -> (date/time string=w606:string)  [unwired: 1 in]
        n315 = case shown="\"MATH\"" w614 {
          tunnel: w613 -> [_ w624 w744]
          tunnel: w611 -> [_ w621 w745]
          tunnel: w609 -> [w617 w620 w741]
          tunnel: [w617 w619 w742] -> w610
          tunnel: w606 -> [_ w618 w743]
          frame Default {
          }
          frame "HAL" {
            n316 = Match Pattern(string=w624, regular expression=":") -> (before substring=w623:string, after substring=w622:string)  [unwired: 1 in, 2 out]
            n317 = case shown="\"HWSync1\"" w623 {
              tunnel: w622 -> [_ w628 w642 w658 w670 w684 w699 w703 w707 w711 w715 w719 w723 w727 w731 w735]
              tunnel: w621 -> [_ w635 w648 w663 w677 w691 _ _ _ _ _ _ _ _ _ _]
              tunnel: w620 -> [w626 w634 w646 w661 w674 w690 w697 w701 w705 w709 w713 w717 w721 w725 w729 w733]
              tunnel: [w626 w633 w647 w660 w675 w689 w697 w701 w705 w709 w713 w717 w721 w725 w729 w733] -> w619
              tunnel: w618 -> [_ w627 w641 w655 w669 w683 _ _ _ _ _ _ _ _ _ _]
              frame "False", Default {
              }
              frame "HWSync1" {
                n318 = Unbundle By Name(w634) -> ("HWS1"=w629:string)
                n319 = Match Pattern(string=w628, regular expression=":") -> (before substring=w631:string)  [unwired: 1 in, 3 out]
                n320 = case shown="\"Digital Out Write\"" w631 {
                  tunnel: w635 -> [_ w640]
                  frame "False", Default {
                  }
                  frame "Digital Out Write" {
                    n321 = Variant To Data(type=0, Variant=w640) -> (data=w638:i32)  [unwired: 1 in, 1 out]
                    n322 = Number To Boolean Array(number=w638) -> (Boolean array=→"DO 1":bool[])
                  }
                }
                n323 = Concatenate Strings(w629, w627, w628, "\r\n") -> (w632:string)
                "HWSync 1" <- w632
                n324 = Bundle By Name(cluster=w634, "HWS1"=w632) -> (w633:T6)
              }
              frame "HWSync2" {
                n325 = Unbundle By Name(w646) -> ("HWS2"=w644:string)
                n326 = Match Pattern(string=w642, regular expression=":") -> (before substring=w649:string)  [unwired: 1 in, 3 out]
                n327 = case shown="\"Digital Out Write\"" w649 {
                  tunnel: w648 -> [_ w654]
                  frame "False", Default {
                  }
                  frame "Digital Out Write" {
                    n328 = Variant To Data(type=0, Variant=w654) -> (data=w652:i32)  [unwired: 1 in, 1 out]
                    n329 = Number To Boolean Array(number=w652) -> (Boolean array=→"DO 2":bool[])
                  }
                }
                n330 = Concatenate Strings(w644, w641, w642, "\r\n") -> (w643:string)
                "HWSync 2" <- w643
                n331 = Bundle By Name(cluster=w646, "HWS2"=w643) -> (w647:T6)
              }
              frame "HWSync3" {
                n332 = Unbundle By Name(w661) -> ("HWS3"=w657:string)
                n333 = Match Pattern(string=w658, regular expression=":") -> (before substring=w662:string)  [unwired: 1 in, 3 out]
                n334 = case shown="\"Digital Out Write\"" w662 {
                  tunnel: w663 -> [_ w668]
                  frame "False", Default {
                  }
                  frame "Digital Out Write" {
                    n335 = Variant To Data(type=0, Variant=w668) -> (data=w666:i32)  [unwired: 1 in, 1 out]
                    n336 = Number To Boolean Array(number=w666) -> (Boolean array=→"DO 3":bool[])
                  }
                }
                n337 = Concatenate Strings(w657, w655, w658, "\r\n") -> (w656:string)
                "HWSync 3" <- w656
                n338 = Bundle By Name(cluster=w661, "HWS3"=w656) -> (w660:T6)
              }
              frame "HWSync4" {
                n339 = Unbundle By Name(w674) -> ("HWS4"=w672:string)
                n340 = Match Pattern(string=w670, regular expression=":") -> (before substring=w676:string)  [unwired: 1 in, 3 out]
                n341 = case shown="\"Digital Out Write\"" w676 {
                  tunnel: w677 -> [_ w682]
                  frame "False", Default {
                  }
                  frame "Digital Out Write" {
                    n342 = Variant To Data(type=0, Variant=w682) -> (data=w680:i32)  [unwired: 1 in, 1 out]
                    n343 = Number To Boolean Array(number=w680) -> (Boolean array=→"DO 4":bool[])
                  }
                }
                n344 = Concatenate Strings(w672, w669, w670, "\r\n") -> (w671:string)
                "HWSync 4" <- w671
                n345 = Bundle By Name(cluster=w674, "HWS4"=w671) -> (w675:T6)
              }
              frame "HWSync5" {
                n346 = Unbundle By Name(w690) -> ("HWS5"=w686:string)
                n347 = Match Pattern(string=w684, regular expression=":") -> (before substring=w688:string)  [unwired: 1 in, 3 out]
                n348 = case shown="\"Digital Out Write\"" w688 {
                  tunnel: w691 -> [_ w696]
                  frame "False", Default {
                  }
                  frame "Digital Out Write" {
                    n349 = Variant To Data(type=0, Variant=w696) -> (data=w694:i32)  [unwired: 1 in, 1 out]
                    n350 = Number To Boolean Array(number=w694) -> (Boolean array=→"DO 5":bool[])
                  }
                }
                n351 = Concatenate Strings(w686, w683, w684, "\r\n") -> (w685:string)
                "HWSync 5" <- w685
                n352 = Bundle By Name(cluster=w690, "HWS5"=w685) -> (w689:T6)
              }
              frame "HWAsync1" {
                n353 = Match Pattern(string=w699, regular expression=":") -> (before substring=→"HWAsync 1":string)  [unwired: 1 in, 3 out]
              }
              frame "HWAsync2" {
                n354 = Match Pattern(string=w703, regular expression=":") -> (before substring=→"HWAsync 2":string)  [unwired: 1 in, 3 out]
              }
              frame "HWAsync3" {
                n355 = Match Pattern(string=w707, regular expression=":") -> (before substring=→"HWAsync 3":string)  [unwired: 1 in, 3 out]
              }
              frame "HWAsync4" {
                n356 = Match Pattern(string=w711, regular expression=":") -> (before substring=→"HWAsync 4":string)  [unwired: 1 in, 3 out]
              }
              frame "HWAsync5" {
                n357 = Match Pattern(string=w715, regular expression=":") -> (before substring=→"HWAsync 5":string)  [unwired: 1 in, 3 out]
              }
              frame "HWAsync6" {
                n358 = Match Pattern(string=w719, regular expression=":") -> (before substring=→"HWAsync 6":string)  [unwired: 1 in, 3 out]
              }
              frame "HWAsync7" {
                n359 = Match Pattern(string=w723, regular expression=":") -> (before substring=→"HWAsync 7":string)  [unwired: 1 in, 3 out]
              }
              frame "HWAsync8" {
                n360 = Match Pattern(string=w727, regular expression=":") -> (before substring=→"HWAsync 8":string)  [unwired: 1 in, 3 out]
              }
              frame "HWAsync9" {
                n361 = Match Pattern(string=w731, regular expression=":") -> (before substring=→"HWAsync 9":string)  [unwired: 1 in, 3 out]
              }
              frame "HWAsync10" {
                n362 = Match Pattern(string=w735, regular expression=":") -> (before substring=→"HWAsync 10":string)  [unwired: 1 in, 3 out]
              }
            }
          }
          frame "MATH" {
            n363 = case shown="\"Scale Calibrate\"" w744 {
              tunnel: w745 -> [_ w753 w809 w824 w836 _]
              tunnel: ["" ("format string") w748 w806 w823 w831 w837] -> w738
              tunnel: w743 -> [_ w747 w794 w815 w830 w839]
              frame Default {
              }
              frame "Solve" {
                n364 = Variant To Data(type=T24 {"format string"="", "Measurement Index"=[]} ("output cluster"), Variant=w753) -> (data=w751:T24)  [unwired: 1 in, 1 out]
                n365 = Unbundle(w751) -> ("format string"=w750:string, "Measurement Index"=w749:i32[])
                n366 = case shown="\"\"" w750 {
                  tunnel: w749 -> [_ w762 w775 w788]
                  tunnel: ["-" w756 w769 w782] -> w748
                  tunnel: w747 -> [_ w755 w768 w781]
                  frame Default {
                  }
                  frame "" {
                    n367 = Number To Decimal String(number=w762) -> (decimal integer string=w761:string[])  [unwired: 1 in]
                    n368 = for {
                      tunnel: w761 -> [w766] mode=indexing
                      shift-right: [w767] -> w759
                      shift-left: "[ " ("String") -> [w763]
                      n369 = Concatenate Strings(w763, "M" ("string"), w766, " " ("String")) -> (w767:string)
                    }
                    n370 = Concatenate Strings(w755, "Resolver Mediciones -> " ("format string"), w759, "]" ("String")) -> (w756:string)
                  }
                  frame "Relev" {
                    n371 = Number To Decimal String(number=w775) -> (decimal integer string=w774:string[])  [unwired: 1 in]
                    n372 = for {
                      tunnel: w774 -> [w779] mode=indexing
                      shift-right: [w780] -> w772
                      shift-left: "[ " ("String") -> [w776]
                      n373 = Concatenate Strings(w776, "M" ("string"), w779, " " ("String")) -> (w780:string)
                    }
                    n374 = Concatenate Strings(w768, "Resolver Mediciones con relevamiento de Pieza Patron -> " ("format string"), w772, "]" ("String")) -> (w769:string)
                  }
                  frame "Mastering" {
                    n375 = Number To Decimal String(number=w788) -> (decimal integer string=w787:string[])  [unwired: 1 in]
                    n376 = for {
                      tunnel: w787 -> [w792] mode=indexing
                      shift-right: [w793] -> w785
                      shift-left: "[ " ("String") -> [w789]
                      n377 = Concatenate Strings(w789, "M" ("string"), w792, " " ("String")) -> (w793:string)
                    }
                    n378 = Concatenate Strings(w781, "Resolver Mediciones con Mastering -> " ("format string"), w785, "]" ("String")) -> (w782:string)
                  }
                }
              }
              frame "Mastering" {
                n379 = Variant To Data(type=T25 {"MAX(T) or MIN (F)?"=FALSE, "Mastering TDX Index"=[]} ("output cluster"), Variant=w809) -> (data=w808:T25)  [unwired: 1 in, 1 out]
                n380 = Unbundle(w808) -> ("MAX(T) or MIN (F)?"=w800:bool, "Mastering TDX Index"=w807:i32[])
                n381 = Number To Decimal String(number=w807) -> (decimal integer string=w805:string[])  [unwired: 1 in]
                n382 = for {
                  tunnel: w805 -> [w813] mode=indexing
                  shift-right: [w814] -> w803
                  shift-left: "[ " ("String") -> [w810]
                  n383 = Concatenate Strings(w810, "T" ("string"), w813, " " ("String")) -> (w814:string)
                }
                n384 = Select(t="MAXIMO" ("format string"), s=w800, f="MINIMO" ("format string")) -> (s? t:f=w796:string)
                n385 = Format Into String(format string="Tomar %s de los Transductores ->", w796) -> (resulting string=w795:string)  [unwired: 2 in, 1 out]
                n386 = Concatenate Strings(w794, w795, w803, "]" ("String")) -> (w806:string)
              }
              frame "Auto-Zero" {
                n387 = Variant To Data(type=i32[] [] ("Mastering TDX Index"), Variant=w824) -> (data=w816:i32[])  [unwired: 1 in, 1 out]
                n388 = Number To Decimal String(number=w816) -> (decimal integer string=w822:string[])  [unwired: 1 in]
                n389 = for {
                  tunnel: w822 -> [w828] mode=indexing
                  shift-right: [w829] -> w820
                  shift-left: "[ " ("String") -> [w825]
                  n390 = Concatenate Strings(w825, "T" ("string"), w828, " " ("String")) -> (w829:string)
                }
                n391 = Concatenate Strings(w815, "Calcular Zero de los Transductores ->" ("format string"), w820, "]" ("String")) -> (w823:string)
              }
              frame "Relev" {
                n392 = Variant To Data(type=0, Variant=w836) -> (data=w833:i32)  [unwired: 1 in, 1 out]
                n393 = Format Into String(format string="Calcular Relevamiento de Pieza Patron en Transductor T%d", w833) -> (resulting string=w832:string)  [unwired: 2 in, 1 out]
                n394 = Concatenate Strings(w830, w832) -> (w831:string)
              }
              frame "Scale Calibrate" {
                n395 = Concatenate Strings(w839, "Calcular Constantes de calibracion de Balanzas" ("format string")) -> (w837:string)
              }
            }
            n396 = Unbundle By Name(w741) -> ("MATH"=w740:string)
            n397 = Concatenate Strings(w740, w738, "\r\n") -> (w737:string)
            "MATH" <- w737
            n398 = Bundle By Name(cluster=w741, "MATH"=w737) -> (w742:T6)
          }
        }
      }
      frame "EXIT" {
      }
      frame "Init" {
        n399 = invoke on="HWSync 1" class="Str" method="Reinit To Default"(error in=w844) -> (error out=w856:errorcluster)  [unwired: 2 in, 2 out]
        n400 = invoke on="HWSync 2" class="Str" method="Reinit To Default"(error in=w844) -> (error out=w855:errorcluster)  [unwired: 2 in, 2 out]
        n401 = invoke on="HWSync 3" class="Str" method="Reinit To Default"(error in=w844) -> (error out=w854:errorcluster)  [unwired: 2 in, 2 out]
        n402 = invoke on="HWSync 4" class="Str" method="Reinit To Default"(error in=w844) -> (error out=w853:errorcluster)  [unwired: 2 in, 2 out]
        n403 = invoke on="HWSync 5" class="Str" method="Reinit To Default"(error in=w844) -> (error out=w852:errorcluster)  [unwired: 2 in, 2 out]
        n404 = invoke on="DO 1" class="Arr (strict)" method="Reinit To Default"(error in=w844) -> (error out=w851:errorcluster)  [unwired: 2 in, 2 out]
        n405 = invoke on="DO 2" class="Arr (strict)" method="Reinit To Default"(error in=w844) -> (error out=w850:errorcluster)  [unwired: 2 in, 2 out]
        n406 = invoke on="DO 3" class="Arr (strict)" method="Reinit To Default"(error in=w844) -> (error out=w849:errorcluster)  [unwired: 2 in, 2 out]
        n407 = invoke on="DO 4" class="Arr (strict)" method="Reinit To Default"(error in=w844) -> (error out=w848:errorcluster)  [unwired: 2 in, 2 out]
        n408 = invoke on="DO 5" class="Arr (strict)" method="Reinit To Default"(error in=w844) -> (error out=w847:errorcluster)  [unwired: 2 in, 2 out]
        n409 = Merge Errors(w856, w855, w854, w853, w852, w851, w850, w849, w848, w847) -> (w845:errorcluster)
        n410 = invoke on="HWAsync 1" class="Str" method="Reinit To Default"(error in=w845) -> (error out=w866:errorcluster)  [unwired: 2 in, 2 out]
        n411 = invoke on="HWAsync 2" class="Str" method="Reinit To Default"(error in=w845) -> (error out=w865:errorcluster)  [unwired: 2 in, 2 out]
        n412 = invoke on="HWAsync 3" class="Str" method="Reinit To Default"(error in=w845) -> (error out=w864:errorcluster)  [unwired: 2 in, 2 out]
        n413 = invoke on="HWAsync 4" class="Str" method="Reinit To Default"(error in=w845) -> (error out=w863:errorcluster)  [unwired: 2 in, 2 out]
        n414 = invoke on="HWAsync 5" class="Str" method="Reinit To Default"(error in=w845) -> (error out=w862:errorcluster)  [unwired: 2 in, 2 out]
        n415 = invoke on="HWAsync 6" class="Str" method="Reinit To Default"(error in=w845) -> (error out=w861:errorcluster)  [unwired: 2 in, 2 out]
        n416 = invoke on="HWAsync 7" class="Str" method="Reinit To Default"(error in=w845) -> (error out=w860:errorcluster)  [unwired: 2 in, 2 out]
        n417 = invoke on="HWAsync 8" class="Str" method="Reinit To Default"(error in=w845) -> (error out=w859:errorcluster)  [unwired: 2 in, 2 out]
        n418 = invoke on="HWAsync 9" class="Str" method="Reinit To Default"(error in=w845) -> (error out=w858:errorcluster)  [unwired: 2 in, 2 out]
        n419 = invoke on="HWAsync 10" class="Str" method="Reinit To Default"(error in=w845) -> (error out=w857:errorcluster)  [unwired: 2 in, 2 out]
        n420 = invoke on="MATH" class="Str" method="Reinit To Default"(error in=w845) -> (error out=w846:errorcluster)  [unwired: 2 in, 2 out]
        n421 = Merge Errors(w866, w865, w864, w863, w862, w861, w860, w859, w858, w857, w846) -> (w843:errorcluster)
      }
      frame "CONFIG" {
        # "\"CONFIG:<Tipo>:<Indice>\" ; <Config Data>"
        n422 = Generate User Event(user event=w871, event data cluster=w872, error in=w870) -> (error out=w869:errorcluster)  [unwired: 1 in, 1 out]
      }
    }
  }
  n423 = while {
    tunnel: w51 -> [w916]
    tunnel: w83 -> [w911]
    tunnel: w81 -> [w909]
    stop <- w910 continue-if-true
    w907 = 200  # Timeout(ms)
    n424 = global read "SEQ Monitoring Global Variables.vi" "Current Sequence"() -> (w880:T4)
    n425 = global read "SEQ Monitoring Global Variables.vi" "Current STEP"() -> (w890:refnum<class "STEP.lvclass">)
    n426 = global read "DO Monitoring Global Variables.vi" "View Out"() -> (→"View Out":T3)
    n427 = global read "DO Monitoring Global Variables.vi" "View Out 2"() -> (→"View Out 2":T3)
    n428 = global read "DO Monitoring Global Variables.vi" "View Out 3"() -> (→"View Out 3":T3)
    n429 = global read "DO Monitoring Global Variables.vi" "View Out 4"() -> (→"View Out 4":T3)
    n430 = global read "DO Monitoring Global Variables.vi" "View Out 5"() -> (→"View Out 5":T3)
    n431 = Wait on Notification(notifier=w916, timeout in ms (-1)=w907, error in (no error)=w911) -> (notification=w908:T8, timed out?=w915:bool, error out=w913:errorcluster)  [unwired: 1 in, 1 out]
    n432 = Wait on Occurrence(1:FALSE ("ignore previous (T)"), 2:w909, 3:w907) -> (0:w910:bool)
    n433 = call <vilib>:"Clear Errors.vi"("error in (no error)"=w913) -> ()  [unwired: 5 in, 2 out]
    n434 = Unbundle By Name(w880) -> ("Main Error&Alarm"=w873:T26, "STEPs"=w879:refnum<class "STEP.lvclass">[])
    n435 = feedback #2(w908) -> (w914:T8)
    n436 = Select(t=w914, s=w915, f=w908) -> (s? t:f=w900:T8)
    n437 = feedback-in #2(w900) -> ()
    n438 = Unbundle By Name(w900) -> ("Mimic Data"=w903:T9, "Operator Mssg"=→"Operator Message":string)
    n439 = Unbundle By Name(w900) -> ("Error.true?"=w881:bool, "Error.Message"=→"Error Message":string)
    "Error" <- w881
    n440 = Unbundle By Name(w900) -> ("Alarm 1"=w899:cluster{"true?":bool, "Message":string}, "Alarm 2"=w898:cluster{"true?":bool, "Message":string}, "Alarm 3"=w897:cluster{"true?":bool, "Message":string}, "Alarm 4"=w896:cluster{"true?":bool, "Message":string})
    n441 = Search 1D Array(1D array=w879, element=w890) -> (index of element=w889:i32)  [unwired: 1 in]
    n442 = for {
      tunnel: w879 -> [w948] mode=indexing
      tunnel: [w947] -> w874 mode=indexing
      n443 = call "Read All Strings.vi"("STEP in"=w948) -> ("All Strings"=w947:string[])  [unwired: 8 in, 2 out]
    }
    n444 = Build Array(w899, w898, w897, w896) -> (w895:cluster{"true?":bool, "Message":string}[])
    n445 = feedback #3(w889) -> (w892:i32)
    n446 = Equal?(x=w892, y=w889) -> (x = y?=w891:bool)
    n447 = feedback-in #3(w889) -> ()
    n448 = for {
      tunnel: w895 -> [w955] mode=indexing
      tunnel: [w950] -> w894 mode=indexing if=w949
      tunnel: [w949] -> w883 mode=indexing
      i -> [w953]
      n449 = Unbundle By Name(w955) -> ("Message"=w951:string, "true?"=w949:bool)
      n450 = Increment(x=w953) -> (x+1=w952:i32)
      n451 = Format Into String(format string="Alarma %d: %s\n", w952, w951) -> (resulting string=w950:string)  [unwired: 2 in, 1 out]
    }
    n452 = case shown="False" w891 {
      tunnel: w889 -> [w930 _]
      frame False {
        n453 = flat-sequence {
          tunnel: w930 -> [w937]
          tunnel: [w937] -> w932
          tunnel: [w934] -> w931
          tunnel: w930 -> [w934]
          tunnel: w932 -> [w943]
          tunnel: w931 -> [w942]
          frame #0 {
            w933 = T13 {"Row"=-2, "Column"=-2} ("Active Cell:Active Cell")
            n454 = property on="Cond. Avan." class="Tbl (strict)"("Active Cell"=w933, "Cell BG Color"=u32 16448250) -> ()  [unwired: 2 in, 2 out]
            n455 = property on="Current Sequence" class="Tbl (strict)"("Active Cell"=w933, "Cell BG Color"=u32 16448250) -> ()  [unwired: 2 in, 2 out]
          }
          frame #1 {
            w938 = cluster{i32, "Row":i32} {0, "Row"=0} ("output cluster")
            n456 = Bundle(cluster=w938, w943, "Row"=-2) -> (w945:cluster{i32, "Row":i32})
            n457 = Bundle(cluster=w938, w942, "Row"=-2) -> (w940:cluster{i32, "Row":i32})
            n458 = property on="Cond. Avan." class="Tbl (strict)"("Active Cell"=w940, "Cell BG Color"=u32 4110335) -> ()  [unwired: 2 in, 2 out]
            n459 = property on="Current Sequence" class="Tbl (strict)"("Active Cell"=w945, "Cell BG Color"=u32 4110335) -> ()  [unwired: 2 in, 2 out]
          }
        }
        n460 = invoke on="Angle" class="Knob (strict)" method="Reinit To Default"() -> ()  [unwired: 3 in, 3 out]
      }
      frame True {
      }
    }
    n461 = feedback #4(w874) -> (w878:string[][])
    n462 = feedback-in #4(w874) -> ()
    n463 = Flatten To String(anything=w878) -> (data string=w877:string)  [unwired: 3 in, 2 out]
    n464 = Flatten To String(anything=w874) -> (data string=w876:string)  [unwired: 3 in, 2 out]
    n465 = property on="Error Message" class="Str"("Blinking"=w881, "Visible"=w881) -> ()  [unwired: 2 in, 2 out]
    n466 = Equal?(x=w877, y=w876) -> (x = y?=w875:bool)
    n467 = case shown="False" w875 {
      tunnel: w874 -> [w927 _]
      tunnel: w873 -> [w923 _]
      frame False {
        n468 = Unbundle By Name(w923) -> ("Main Error.Formula"=w921:string, "Main Alarm 1.Formula"=w920:string, "Main Alarm 2.Formula"=w922:string, "Main Alarm 3.Formula"=w919:string, "Main Alarm 4.Formula"=w918:string)
        n469 = Build Array(w921, w920, w922, w919, w918) -> (w917:string[])
        n470 = Insert Into Array(array=string[][] [] ("Show Main Error&Alarm 2"), index (row)=0, new element=w917) -> (→"Show Main Error&Alarm":string[][])  [unwired: 1 in]
        n471 = Delete From Array(array=w927, index (col)=0 ("disabled index (col)")) -> (array with subset deleted=→"Cond. Avan.":string[][])  [unwired: 2 in, 1 out]
        "Current Sequence" <- w927
      }
      frame True {
      }
    }
    n472 = call "Draw Mimic Image.vi"("Mimic Data in"=w903) -> ("Mimic Picture"=w906:picture)  [unwired: 10 in]
    "Mimic" <- w906
    "Mimic Small" <- w906
    n473 = Or Array Elements(Boolean array=w883) -> (logical OR=→"Alarma":bool)
    n474 = Concatenate Strings(w894) -> (→"Alarms Message":string)
    n475 = control-ref of="Mimic"() -> (w905:refnum<vi>)
    n476 = control-ref of="Mimic Small"() -> (w904:refnum<vi>)
    n477 = call "Fit Image to Ctrl (SubVI).vi"("picture in"=w906, "Picture ref in"=w905) -> ()  [unwired: 10 in]
    n478 = call "Fit Image to Ctrl (SubVI).vi"("picture in"=w906, "Picture ref in"=w904) -> ()  [unwired: 10 in]
  }
  n479 = call "SeqLoop.vi"("SEQ STEP Display"=w51, "error in (no error)"=w56, "SEQ"=w58, "CORE"=w59, "WINFAS 2 Data Queue"=w57) -> ("error out"=w55:errorcluster)  [unwired: 6 in]
  n480 = Set Occurrence(w82) -> ()
  n481 = Merge Errors(w101, w55) -> (w98:errorcluster)
  n482 = call "Destroy All Message Queues.vi"("error in (no error)"=w98, "Message Queues Out"=w61) -> ("error out"=w63:errorcluster)  [unwired: 9 in]
  n483 = call "Destroy All Data Queues.vi"("Error In"=w63, "WINFAS 2 Data Queue.lvlib:All Data Queues Cluster"=w57) -> ("Error Out"=w62:errorcluster)  [unwired: 9 in]
  n484 = Release Notifier(notifier=w51, error in (no error)=w62) -> (error out=w84:errorcluster)  [unwired: 1 in, 2 out]
  n485 = property class="App"(error in=w84) -> ("App.Kind"=w89:T27)  [unwired: 1 in, 2 out]
  n486 = case shown="\"Run Time System\"" w89 {
    tunnel: [TRUE FALSE TRUE] -> w88
    tunnel: [w956 w970 w976] -> _
    frame "invalid app kind", Default {
      n487 = property class="VI"() -> (error out=w957:errorcluster, "Panel"=w967:refnum<vi>)  [unwired: 2 in, 1 out]
      n488 = property class="Pnl"(reference=w967, error in=w957) -> (error out=w958:errorcluster, "AllObjs[]"=w966:refnum<vi>[])  [unwired: 1 out]
      n489 = control-ref of="This VI"() -> (w964:refnum<vi>)
      n490 = Close Reference(reference=w966, error in (no error)=w958) -> (error out=w963:errorcluster)
      n491 = invoke class="VI" method="FP.Close"(reference=w964, error in=w963) -> (reference out=w962:refnum<vi>, error out=w961:errorcluster)  [unwired: 1 in, 1 out]
      n492 = invoke class="VI" method="Abort VI"(reference=w962, error in=w961) -> (reference out=w959:refnum<vi>, error out=w960:errorcluster)  [unwired: 1 in, 1 out]
      n493 = Close Reference(reference=w959, error in (no error)=w960) -> (error out=w968:errorcluster)
      n494 = control-ref of="This Application"() -> (w969:refnum<vi>)
      n495 = Close Reference(reference=w969, error in (no error)=w968) -> (error out=w956:errorcluster)
    }
    frame "Development System" {
      n496 = property class="VI"() -> (error out=w971:errorcluster, "Panel"=w975:refnum<vi>)  [unwired: 2 in, 1 out]
      n497 = property class="Pnl"(reference=w975, error in=w971) -> (error out=w972:errorcluster, "AllObjs[]"=w974:refnum<vi>[])  [unwired: 1 out]
      n498 = Close Reference(reference=w974, error in (no error)=w972) -> (error out=w970:errorcluster)
    }
    frame "Run Time System" {
      n499 = property class="VI"() -> (error out=w977:errorcluster, "Panel"=w987:refnum<vi>)  [unwired: 2 in, 1 out]
      n500 = property class="Pnl"(reference=w987, error in=w977) -> (error out=w978:errorcluster, "AllObjs[]"=w986:refnum<vi>[])  [unwired: 1 out]
      n501 = control-ref of="This VI"() -> (w984:refnum<vi>)
      n502 = Close Reference(reference=w986, error in (no error)=w978) -> (error out=w983:errorcluster)
      n503 = invoke class="VI" method="FP.Close"(reference=w984, error in=w983) -> (reference out=w982:refnum<vi>, error out=w981:errorcluster)  [unwired: 1 in, 1 out]
      n504 = invoke class="VI" method="Abort VI"(reference=w982, error in=w981) -> (reference out=w979:refnum<vi>, error out=w980:errorcluster)  [unwired: 1 in, 1 out]
      n505 = Close Reference(reference=w979, error in (no error)=w980) -> (error out=w988:errorcluster)
      n506 = control-ref of="This Application"() -> (w989:refnum<vi>)
      n507 = Close Reference(reference=w989, error in (no error)=w988) -> (error out=w976:errorcluster)
    }
  }
  n508 = Quit LabVIEW(quit? (T)=w88) -> ()
